vi "MAIN_8.1.vi"() -> ()   [LabVIEW 2013]
doc: "Use this template to build a producer/consumer design pattern with events to produce queue items. Use this design pattern instead of the User Interface Event Handler pattern for user interfaces when you want to execute code asynchronously in response to an event without slowing the user interface responsiveness."
uses:
  State_machine_enum.ctl
  display2.ctl
  User_buttons_enum.ctl
  <vilib>/Analysis/baseanly.llb/Mean (DBL).vi
  <vilib>/DAQmx/read.llb/DAQmx Read (Analog 2D DBL NChan NSamp).vi
  Global 1_diag.vi
  <vilib>/Waveform/WDTFileIO.llb/Export Waveforms To Spreadsheet File (1D).vi
  <vilib>/Utility/file.llb/Write To Spreadsheet File (DBL).vi
  <vilib>/Waveform/WDTFileIO.llb/Export Waveform To Spreadsheet File.vi
  <vilib>/DAQmx/create/channels.llb/DAQmx Create Channel (AI-Voltage-Basic).vi
  <vilib>/DAQmx/configure/timing.llb/DAQmx Timing (Sample Clock).vi
  <vilib>/DAQmx/miscellaneous.llb/DAQmx Fill In Error Info.vi
  <vilib>/express/express arith-compare/Formula/XNode/ExpressFormulaBlockNode.xnode
  <vilib>/Analysis/NI_AALBase.lvlib
  <resource>/objmgr/daqmx.rc
panel:
  out "1f PEM Y":dbl
  out "2f PEM Y":dbl=0.004981012167818904
  out "2f PEM X":dbl=0.004981012167818904
  out "1f PEM X":dbl
  out "2f Spectrum array":dbl[](array[numeric])
  in  "QuickDiag":bool=TRUE
  out "x/y":dbl=0.002005684477504462
  in  "Motor Voltage (V) 2":dbl=1.0 min=0.0 max=9.0
  in  "Time Resolved":bool=TRUE
  in  "Start time":timestamp=timestamp(-9593251199.274853 s since 1904-01-01)
  in  "Timer Start":bool
  out "path":path=path "C:/Users/Adam/Desktop/Diag_Prog_v9/temp.txt"
  in  "Stabilization Time (s)":dbl min=0.0 max=2.0
  out "LD error array disc":dbl[](array[numeric])
  out "LD array disc":dbl[](array[numeric])
  out "result":bool=TRUE
  out "dt":dbl=0.001
  out "dLD_RMS":dbl=-0.0
  out "error out":errorcluster
  out "Unbalanced?":bool
  out "Signal Balance":bool
  out "DC Voltage (V) 2":dbl(knob)=0.000879695520089483 scale=0.0..10.0
  out "2f Frequency (Hz)":dbl(knob)=512.4961246512186 scale=0.0..150.0
  in  "Voltage Divider (10)":bool
  out "Actual Task":string="Processing signal"
  out "Motor Voltage (V)":dbl=1.0
  in  "Initial Voltage (V)":dbl=0.35 min=0.0 max=9.0
  in  "Final Voltage (V)":dbl=0.8 min=0.0 max=2.0
  in  "Voltage Step (V)":dbl=0.065 min=0.0 max=1000.0
  in  "Motor Stabilization Time (s)":dbl(knob)=10.0 step=0.001 scale=0.0..30.0
  out "Initial Voltage (V) 2":dbl=1.0 min=0.0 max=9.0
  in  "Final Voltage (V) 2":dbl=1.4 min=0.0 max=2.0
  in  "Voltage Step (V) 2":dbl=0.1 min=0.0 max=1000.0
  in  "Comment (sample no)":string
  in  "Stop Measurement":bool
  in  "Start Measurement Button":bool
  out "Measurement File":path=path "C:/Users/Adam/Desktop/Diag_Prog_v9/testt"
  in  "New File":bool
  out "Reset?":bool=TRUE
  out "Actual State":T1=enum."Process"
  in  "Tab Control":T2(tab)
  out "Measured Points":T3 format="%0.3f"
  out "Ready?":bool
  out "Ready?":string="Ready?"
  out "Motor":bool=TRUE
  out "Motor":string="Motor: OK"
  out "Quick Status 5":string
  out "Down 2":bool
  out "Up 2":bool
  out "Oscilloscope 2":waveform(dbl)[](graph)=[{"t0"=timestamp(0 s since 1904-01-01), "dt"=0.002, "Y"=array[500 elements]}, {"t0"=timestamp(0 s since 1904-01-01), "dt"=0.002, "Y"=array[500 elements]}]
  out "Signal Balance":bool=TRUE
  out "Laser Noise":bool=TRUE
  out "Signal Balance":string="Signal Balance: OK"
  out "Laser Noise":string="Laser Noise: OK"
  in  "Run Quick Diagnostics":bool
  out "Laser Intensity":bool=TRUE
  out "Laser Intensity":string="Laser Intensity: OK"
  out "Delta":T3 format="%0.3f"
  out "Quick Diagnosis":string="?"
  out "Infected?":bool
  out "Detected Signal (mV/V)":T3 format="%0.3f"
  in  "Measure":bool
  out "Signal Spectrum (mVrms/Vdc) 2":cluster{"f0":dbl, "df":dbl, "magnitude":dbl[]}(graph)={"f0"=0.0, "df"=0.05, "magnitude"=[]}
  in  "Convert mld":bool
  in  "Convert parasiteno":bool
  in  "Convert parasitemia":bool
  in  "Convert cc":bool
  out "MLD (mV/V)":dbl=3.234067345901155 format="%#_3g"
  out "SA 1f (mv/V)":dbl=2.8989130211772483
  out "Lock_in (mV/V)":dbl
  out "dLock_in (mV/V)":dbl
  out "dMLD (mV/V)":dbl=1.4958145805121073 format="%#_3g"
  out "Phase (deg)":dbl=0.5117629371467104 format="%0.2f"
  out "Phase  dev (deg)":dbl=-1.4797919911802346 format="%0.2f"
  out "SA 2f (mv/V)":dbl=4.7886484733621755
  out "MLD Amplitude (mV/V)":cluster{dbl[], dbl[]}(graph)={[811.3544417222341, 811.3544417222341, 811.3544417222341, 812.123069024086, 812.123069024086, 812.123069024086, 812.8874794085821, 812.8874794085821, 812.8874794085821], [1.2454269974542926, 0.5310286252314307, nan, 2.0283944559953087, 0.629318419816088, nan, 4.729881926413262, 1.7382527653890476, nan]}
  in  "dT/T (%)":dbl
  in  "Dilution":dbl=20.0
  in  "Undiluted cc.\n (ng/ml)":dbl
  in  "Undiluted \nParasitemia (%)":dbl format="%#_6f"
  in  "Parasites/ul\nof Blood":dbl
  in  "Convert dT":bool
  in  "MLD (mV/V)":dbl
  out "mean MLD (mV/V)":T3 format="%0.3f"
  out "Delta MLD":T3 format="%0.3f"
  out "DC (V)":cluster{dbl[], dbl[]}(graph)={[811.3544417222341, 812.123069024086, 812.8874794085821], [0.0013390360406046716, 0.001032809026927879, 0.0011348846981534767]}
  out "MLD Phase":cluster{dbl[], dbl[]}(graph)={[811.3544417222341, 811.3544417222341, 811.3544417222341, 812.123069024086, 812.123069024086, 812.123069024086, 812.8874794085821, 812.8874794085821, 812.8874794085821], [3.334514079178165, 1.9138777094600323, nan, 1.9127445130109195, 0.49437453619101257, nan, nan, nan, nan]}
  out "Down":bool
  out "Up":bool
  out "2f Frequency (Hz)":T3=23.056300268096514 format="%0.3f"
  out "1f SA (mV/V)":T3=153.49895465158366 format="%0.3f"
  out "MLD Sim. LIA (mV/V)":T3=nan format="%0.3f"
  out "MLD SA (mV/V)":T3=37.38207236557522 format="%0.3f"
  in  "Start Scope":bool
  in  "Constant Motor Voltage":dbl=1.0 min=0.0 max=3.0
  in  "Refresh in (s)":i8=10
  in  "stop":bool
  in  "AC?":bool
  out "levelB":dbl=0.1 format="%#_2g"
  out "levelA":dbl format="%#_3g"
  in  "V/div B":dbl(knob)=0.2 scale=10.0..0.01 scale format="%#_3g"
  in  "level B":dbl(slide)=0.4 scale=-1.0..1.0 scale format="%#_3g"
  in  "level A":dbl(slide) scale=-1.0..1.0 scale format="%#_3g"
  in  "V/div A":dbl(knob)=0.05 scale=10.0..0.01 scale format="%#.3f"
  out "Oscilloscope":waveform(dbl)[](graph)=[{"t0"=timestamp(0 s since 1904-01-01), "dt"=0.0025, "Y"=array[375 elements]}, {"t0"=timestamp(0 s since 1904-01-01), "dt"=0.0025, "Y"=array[375 elements]}]
  in  "Sensitivity":T4(ring)
  in  "samples per channel":i32=1000
  in  "rate":dbl=1000.0 format="%0.2f"
  out "Spectrum (mVRMS/Vdc)":cluster{"f0":dbl, "df":dbl, "magnitude":dbl[]}(graph)={"f0"=0.0, "df"=1.0, "magnitude"=[1338.0484216778725, 891.4717650116102, 143.2192215595614, 172.79898091711885, 95.50453001628563, 113.23096269717587, 159.9728459536367, 142.17510842649094, 23.555096842939967, 172.4586840116519, 233.3391086271948, 153.49895465158366, 59.303017218056304, 51.41913744169332, 87.60985790792097, 89.15548748523767, 102.41083253503767, 116.69415211742178, 102.04780407888852, 98.07941394008398, 62.015801498942174, 57.365633541451224, 37.38207236557522, 140.01194138717574, 88.85968438008766, 51.8911573784031, 96.44625566359282, 102.80626369349147, 154.32416325374467, 152.72565881880075, 63.97627104136422, 44.061183722532256, 24.299532372372934, 66.51944362511281, 119.45636901763923, 79.60274206424093, 126.46507446936278, 115.56735495111872, 86.92439368676867, 42.47483057858276, 45.987972767001125, 82.38613913097223, 57.14235729256332, 24.715704736492583, 91.95786457200892, 229.45656360476565, 301.7932887816684, 181.94479488218664, 9.707170408716356, 79.16705422107816, 32.4671901662433, 34.994674897672475, 45.603676560961965, 81.17087782317107, 123.48392300390853, 125.53549820312338, 197.71297955832767, 51.56670220175255, 139.4897349387358, 136.00021553543283, 49.84751230386803, 106.388211919061, 128.21302631973177, 179.83380975700697, 238.686425101159, 204.64888147263136, 159.4400865495827, 88.9566203515302, 50.82386237011203, 47.10090178269198, 31.249556983451996, 155.07366739734923, 197.20488460315576, 181.86491698592144, 122.60135896300172, 15.723508058553668, 47.32988919426525, 91.09235604990127, 70.08764782926058, 71.11042986773145, 167.58334514547386, 157.0684001711449, 85.4088975978964, 165.68125229281705, 108.34787076535925, 58.32465184772515, 102.85811162079386, 88.031264754637, 35.99088343784742, 74.99228300753498, 59.59436041355427, 109.74543517855098, 239.92689639368845, 195.22681808589817, 153.93792803433803, 171.35120542643082, 103.04216715301814, 144.22424620891795, 33.236928017526, 33.6474288996255, 71.18496484217899, 175.10446025244616, 221.24997378317522, 114.75466832528755, 52.3833439055373, 114.90211538243959, 94.87498722211751, 82.82924122532899, 124.12586199482064, 107.6258638888207, 78.5024563400891, 92.06245924719637, 16.228987466475928, 84.84217000760313, 88.76503911599063, 114.25618103440272, 155.27289903749065, 116.20062823456668, 61.96139303164934, 214.19314697712042, 248.12058486418763, 215.9112937618697, 145.04293815290015, 142.16464369485132, 169.7377761460246, 83.55657324380019, 74.4879617799582, 39.81106304135121, 152.2410798694005, 176.4879867987291, 110.01229615691923, 89.83888006443468, 195.69702436303007, 166.19892376632072, 55.02836867851484, 113.06515146784245, 221.3685360221306, 181.10055208661387, 262.0371181638539, 185.73443857709046, 93.90961856721144, 84.54783744027858, 24.449872475327695, 95.3789149136639, 140.24246950513043, 143.73337464437884, 33.58378655631947, 62.839362697344995, 57.47449635929643, 139.96968907631262, 167.0231838520772, 135.6723918020847, 124.14523269479409, 111.37946391963057, 195.70470757666732, 192.9947832776428, 93.91006382282066, 121.56931305302999, 113.63589006917633, 42.92804035457153, 141.48803985115433, 165.5507518379778, 121.34962379960878, 143.04362518480343, 22.72432951654588, 183.17549468524615, 152.95042171438013, 195.3079831947777, 131.83171839040367, 30.49881104219535, 8.46043248589554, 141.40803256070282, 223.72992955634092, 132.30059550265176, 54.60897309407436, 84.56504745319246, 125.72411835874722, 194.72474433717994, 126.94182365881618, 27.456941187399302, 114.85067679816903, 138.3914927403539, 237.22038521157256, 172.58040690453, 178.93819766022105, 171.11586449112946, 66.32529189912087, 175.61268977844438, 179.0727535154661, 223.71442469320746, 230.52161416220554, 181.0440521026372, 72.70233235363926, 157.99312186800248, 143.29067791998708, 138.45794114882568, 122.15383561979628, 55.90884824057415, 43.2895289444191, 25.99180252149831]}
  out "MLD LIA (mV/V)":dbl=0.0123978
  out "Lockin_freq":dbl=9.4676
  out "DC Voltage (V)":T3=0.000879695520089483 format="%0.3f"
  out "Time Domain Signal":cluster{"xi used":dbl[], "yi":dbl[]}[](graph)
  out "Signal Spectrum (mVrms/Vdc)":cluster{"f0":dbl, "df":dbl, "magnitude":dbl[]}[](graph)=[{"f0"=0.0, "df"=0.049999500004999954, "magnitude"=array[50001 elements]}, {"f0"=0.0, "df"=0.05, "magnitude"=array[5000 elements]}]
  out "1f 2f Spectral Peaks":T5={"1f (Hz)"=256.112805640282, "U1f (mV/V)"=2.8989130211772483, "2f (Hz)"=512.375618780939, "U2f (mV/V)"=4.7886484733621755}
  out "LockIN Theta (cont/disc)":waveform(dbl)(graph)={"t0"=timestamp(0 s since 1904-01-01), "dt"=0.002, "Y"=array[5000 elements]}
  out "LockIN R (cont/disc)":waveform(dbl)(graph)={"t0"=timestamp(0 s since 1904-01-01), "dt"=0.002, "Y"=array[5000 elements]}
  out "Lockin R":waveform(dbl)(graph)
  out "Lockin Theta":waveform(dbl)(graph)
  out "2f PEM R":dbl=0.004981012167818904
  out "1f PEM R":dbl
  out "PEM spectrum":cluster{"f0":dbl, "df":dbl, "magnitude":dbl[]}(graph)
  out "Lockin X,Y,R":waveform(dbl)[](graph)
  out "PEM spectrum X,Y,R":cluster{"f0":dbl, "df":dbl, "magnitude":dbl[]}[](graph)
  in  "Pike Removal (StDev)":dbl=3.0
  in  "Lock-in Time (s)":dbl=10.0
  in  "dt (s)":dbl=0.0002
  in  "Resolution (s)":dbl=0.0001
  in  "Averaging time (s)":dbl=1.0 format="%0.2p"
  in  "Cutoff Frequency (Hz)":dbl=500.0
  in  "Rate":dbl=5000.0 caption="Sample Rate (Hz)" format="%0.2f"
  in  "Samples per Channel":i32=100000
  out "Minimum Value":dbl=-1.0 caption="LD min Value (V)" format="%0.2f"
  out "Maximum Value":dbl=1.0 caption="LD max Value (V)" format="%0.2f"
  in  "DC # samples":i32=100
  in  "DC Sampling Rate (Hz)":dbl=100.0
  in  "Dc min":dbl format="%0.2f"
  in  "Dc max":dbl=10.0 format="%0.2f"
  in  "Reference Signal":tag="Dev2/ai3"
  in  "LD Signal":tag="Dev2/ai0" caption="LD Channel"
  in  "DC Voltage DAQ":tag="Dev2/ai1"
  in  "Motor Channel":tag="Dev2/ao0"
  in  "Lock-in-Amplifier VISA":refnum<visa-resource-name>="GPIB0::3::INSTR"
  in  "Second Harmonic":bool
  in  "Lock In":bool
  in  "Continous Lock-in":bool=TRUE
  in  "LockIn":bool
  in  "Save graphs":bool
  out "Dc standard deviation":dbl=0.002551891780639937 format="%0.2f"
  out "Dc mean":dbl=0.000879695520089483 format="%0.2f"
  out "dPhase array":dbl[](array[numeric])=[0.7103181848590662, 0.7091849884099535, 0.5117629371467104]
  out "Phase array":dbl[](array[numeric])=[2.6241958943190986, 1.203559524600966, nan, 1.2024263281518537, -0.21594364866805338, nan, -1.4797919911802346]
  out "LD array":dbl[](array[numeric])=[0.8882278113428617, 1.3288564379056984, 3.234067345901155]
  out "Frequency array":dbl[](array[numeric])=[811.3544417222341, 812.123069024086, 812.8874794085821]
  out "LD error array":dbl[](array[numeric])=[0.357199186111431, 0.6995380180896104, 1.4958145805121073]
  out "First?":bool
  out "Stopped":bool
  out "Last Step?":bool
  in  "EXIT":bool
  # "Measurement Settings"
  # "Motor Setup"
  # "OFF"
  # "ON"
  # "Setup"
  # "Status:"
  # "Measurement"
  # "mV/V"
  # "±"
  # "Detected Magneto-Optical Signal:"
  # "Quick Diagnosis Report:"
  # "Measured points:"
  # "Actual Datapoint Values"
  # "mV/V"
  # "±"
  # "Convert quantities"
  # "Physical channels"
  # "Signal Processing Settings"
  # "DC Acquisition Settings"
  # "LD Acquisition Settings"
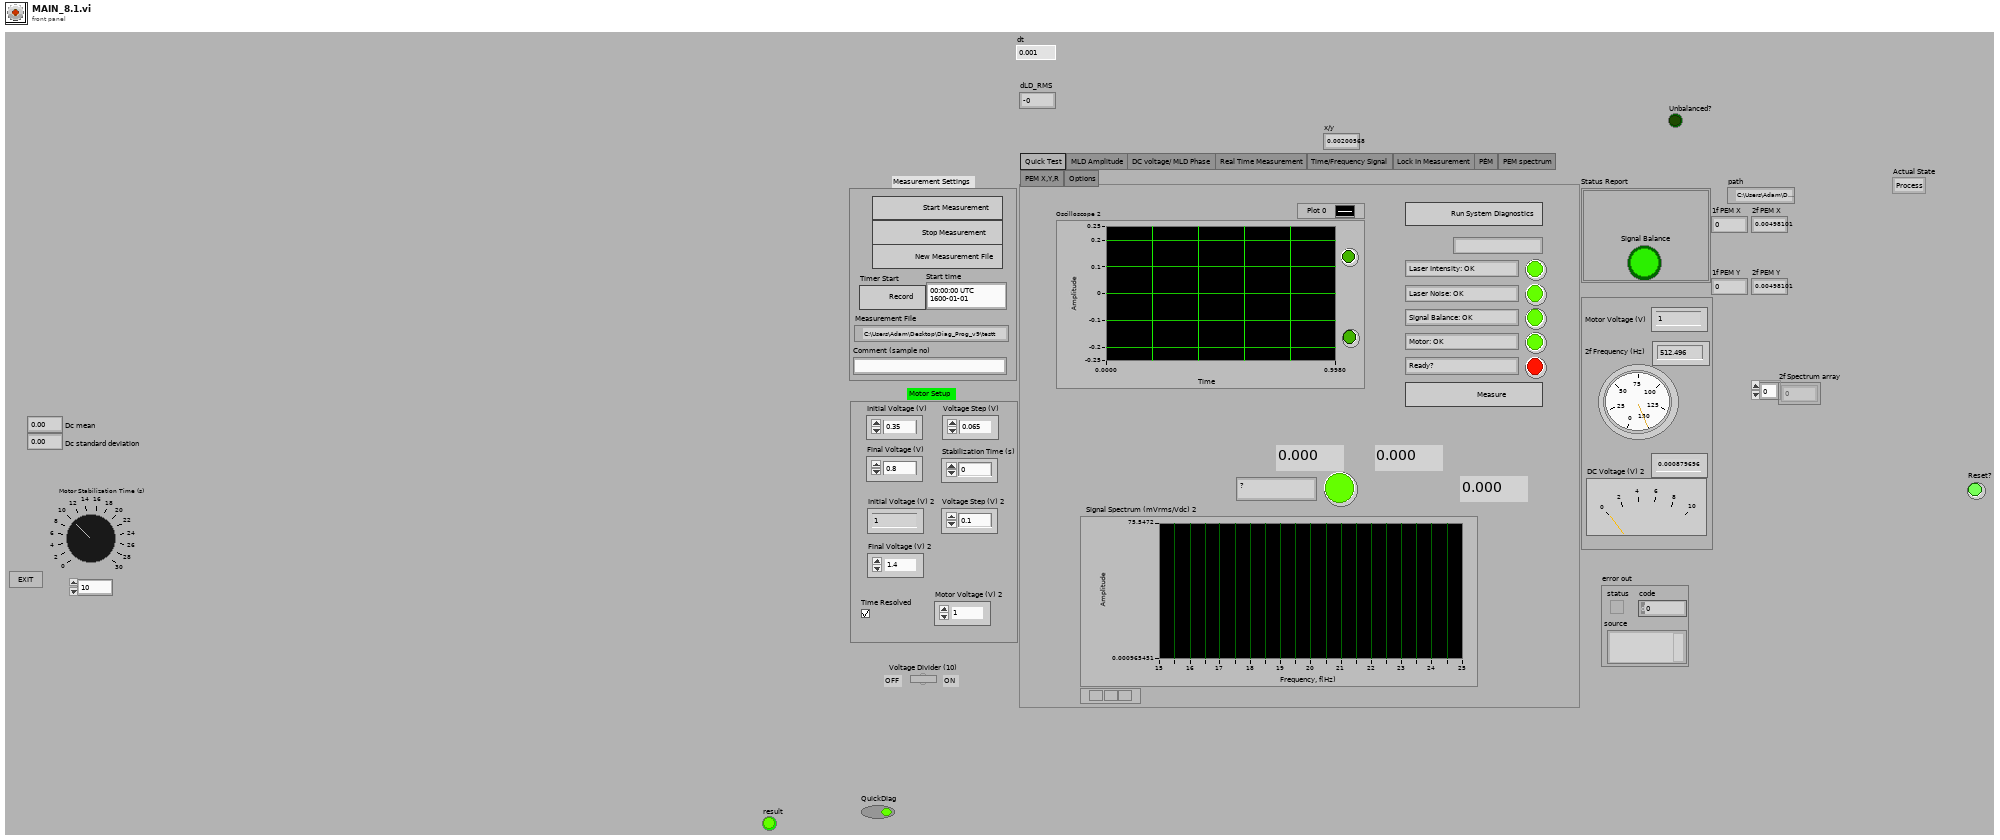
[diagram p1: front panel]
types:
  T1 = typedef "State_machine_enum.ctl" = enum16{"SetMotor", "Stabilize", "Measure", "Process", "Save", "Finished"}
  T2 = enum32{"Quick Test", "MLD Amplitude", "DC voltage/ MLD Phase", "Real Time Measurement", "Time/Frequency Signal", "Lock In Measurement", "PÉM", "PEM spectrum", "PEM X,Y,R", "Options"}
  T3 = typedef "display2.ctl" = dbl
  T4 = enum16{"-1V..1V", "-1.25V..1.25V", "-2V..2V", "-2.5V..2.5V", "-4V..4V", "-5V..5V", "-10V..10V"}
  T5 = cluster{"1f (Hz)":dbl, "U1f (mV/V)":dbl, "2f (Hz)":dbl, "U2f (mV/V)":dbl}
  T6 = typedef "User_buttons_enum.ctl" = enum16{"start", "stop", "exit", "New", "Scope", "Continue"}
  T7 = enum16{"open", "replace", "create", "open or create", "replace or create", "replace or create with confirmation"}
  T8 = enum8{"Enabled", "Disabled", "Disabled and Grayed Out"}
  T9 = enum16{"Left Button", "Center Button", "Right Button", "Window Close"}
  T10 = cluster{dbl, "1f Ampl (Vrms/Vdc)":dbl, dbl, "2f Ampl (Vrms/Vdc)":dbl}
  T11 = cluster{"MLD":dbl, "dMLD":dbl, "Phase":dbl, "dPhase":dbl}
  T12 = cluster{"Frequency array":dbl[], "LD array":dbl[]}
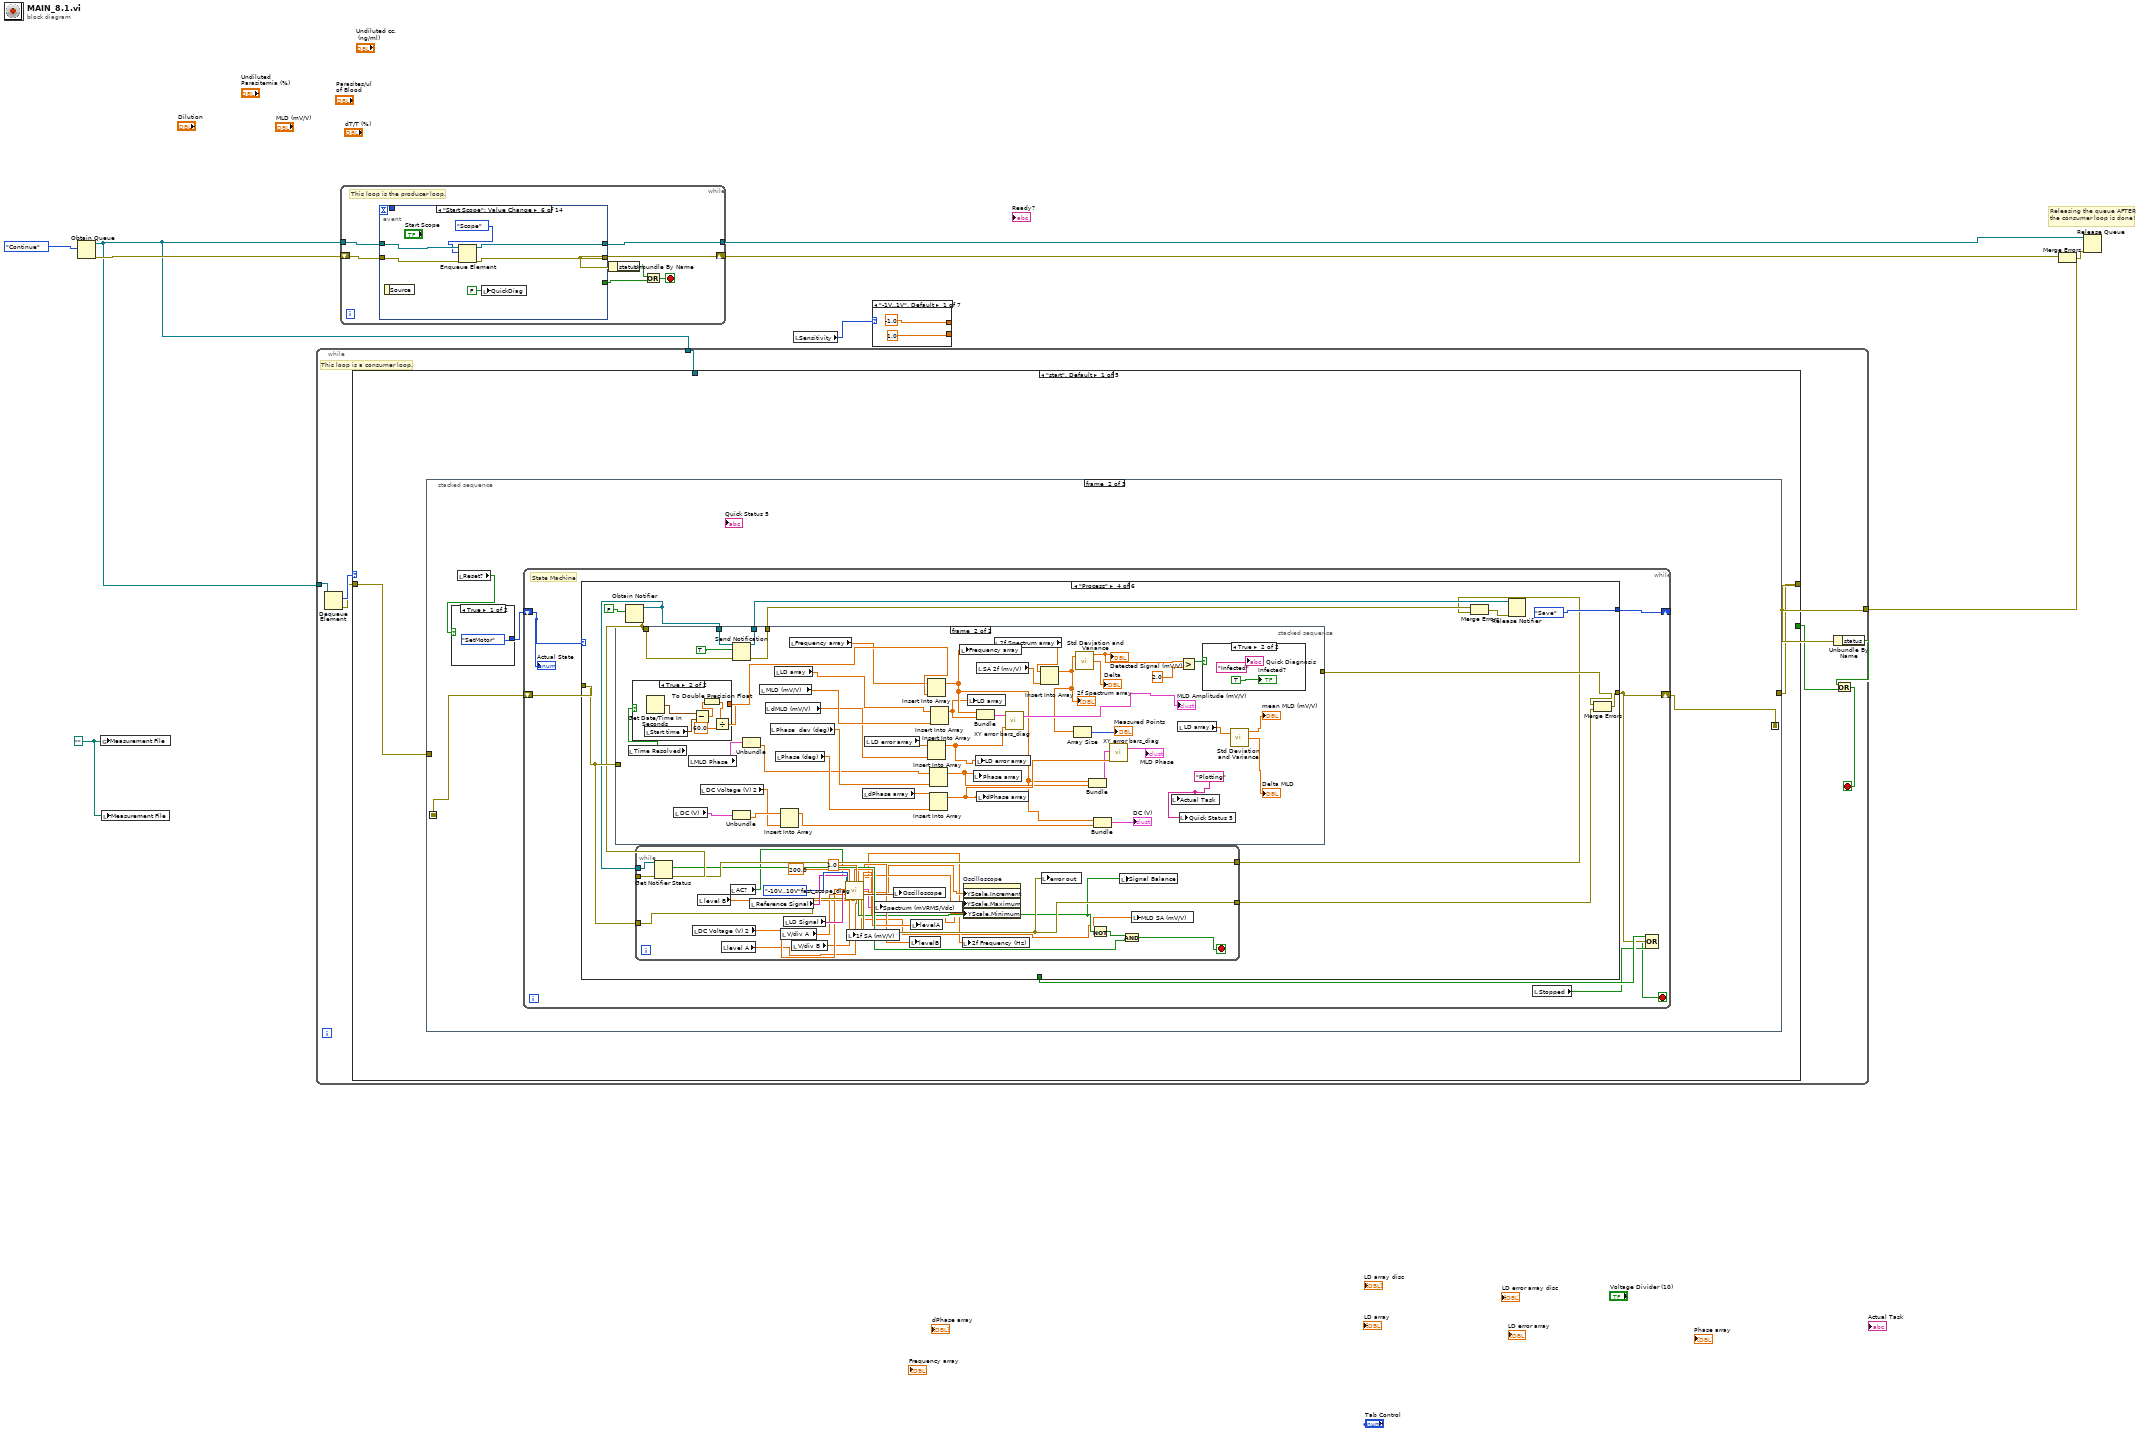
[diagram p0: block diagram]
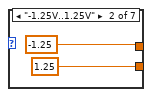
[diagram p2: hidden frame]
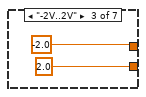
[diagram p3: hidden frame]
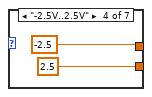
[diagram p4: hidden frame]
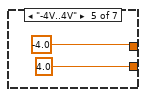
[diagram p5: hidden frame]
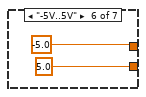
[diagram p6: hidden frame]
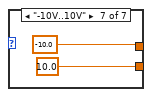
[diagram p7: hidden frame]
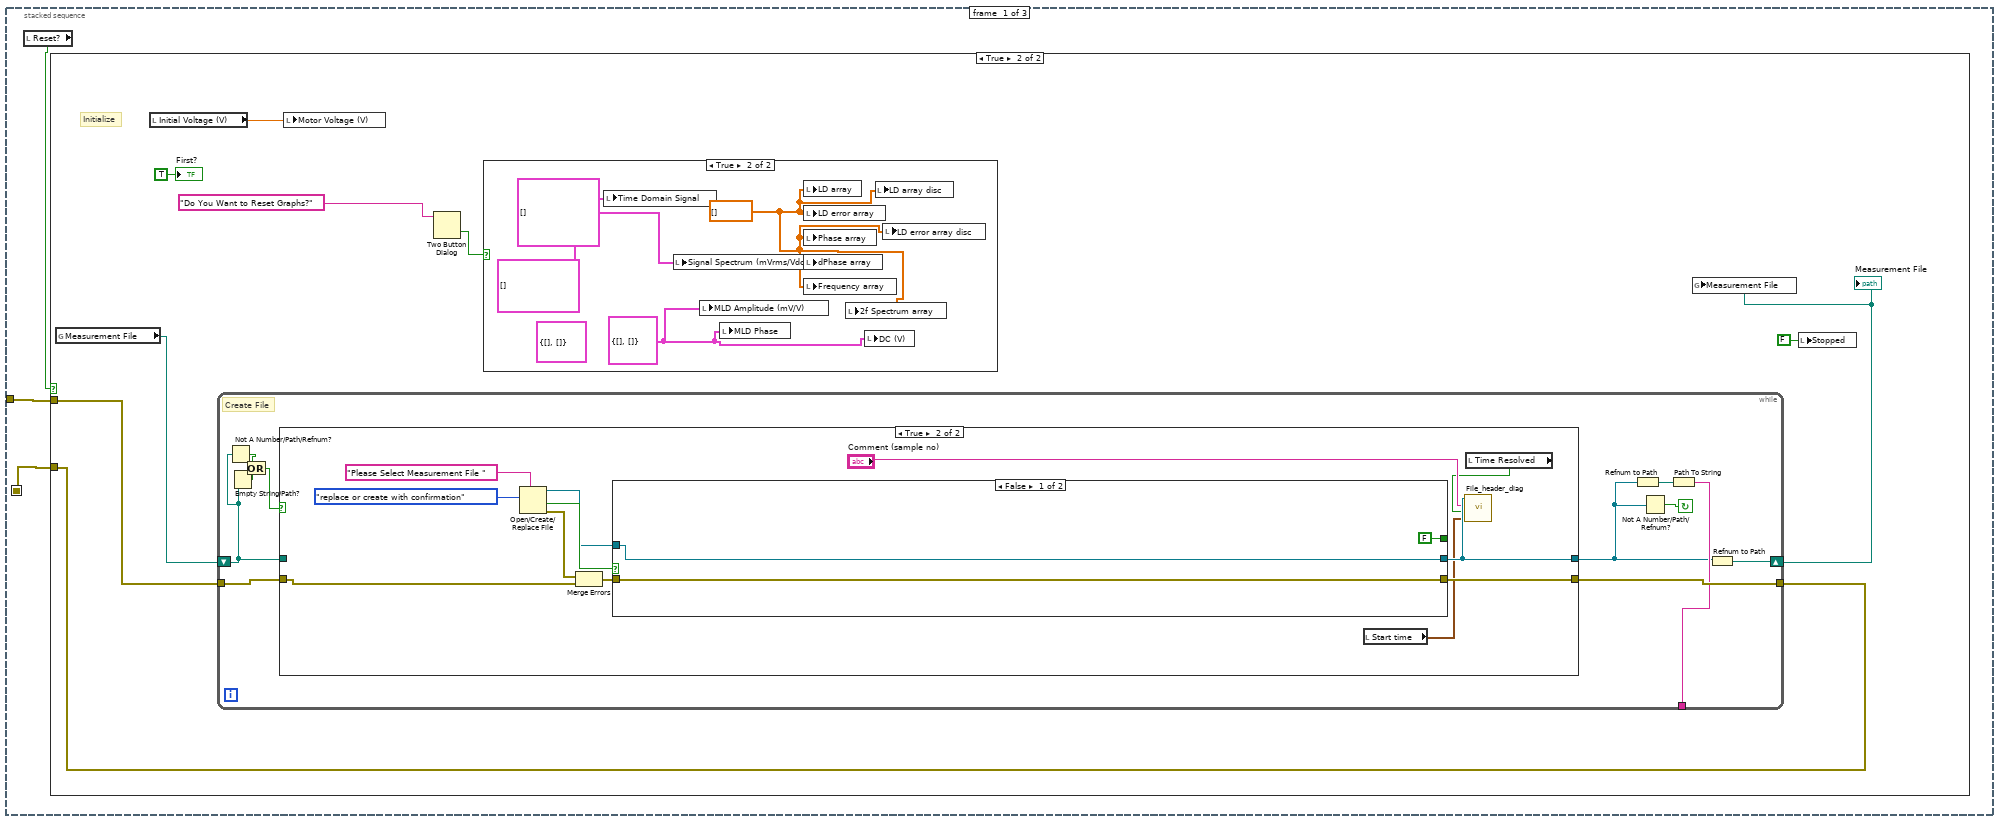
[diagram p8: hidden frame]
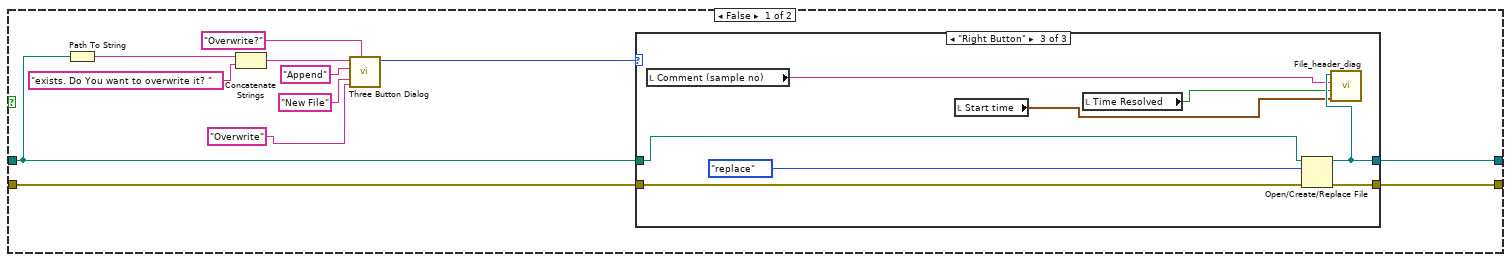
[diagram p10: hidden frame]
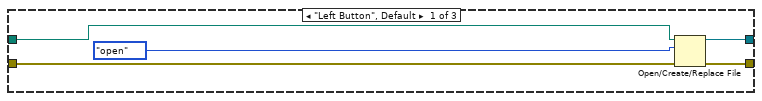
[diagram p11: hidden frame]
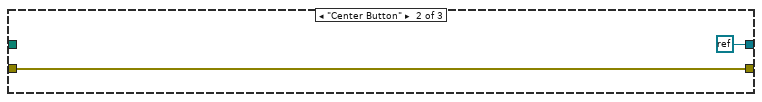
[diagram p12: hidden frame]
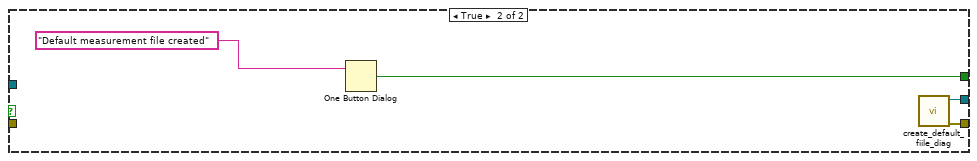
[diagram p13: hidden frame]
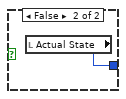
[diagram p15: hidden frame]
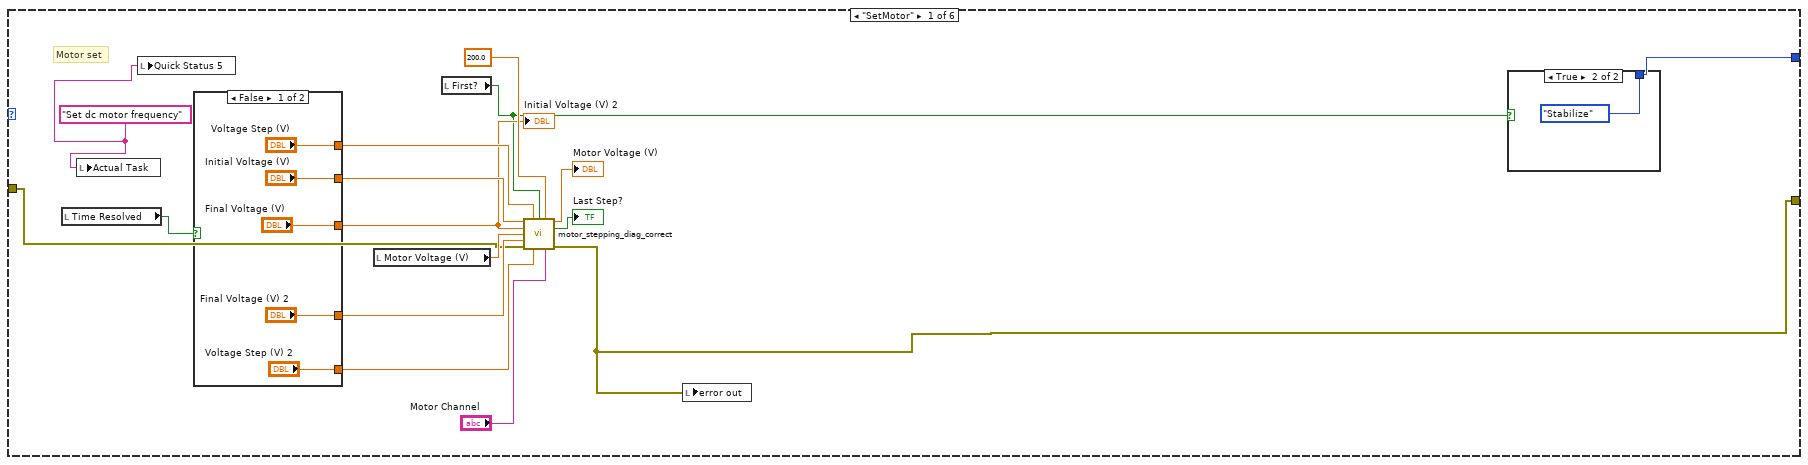
[diagram p16: hidden frame]
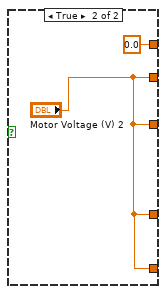
[diagram p17: hidden frame]
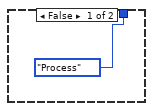
[diagram p18: hidden frame]
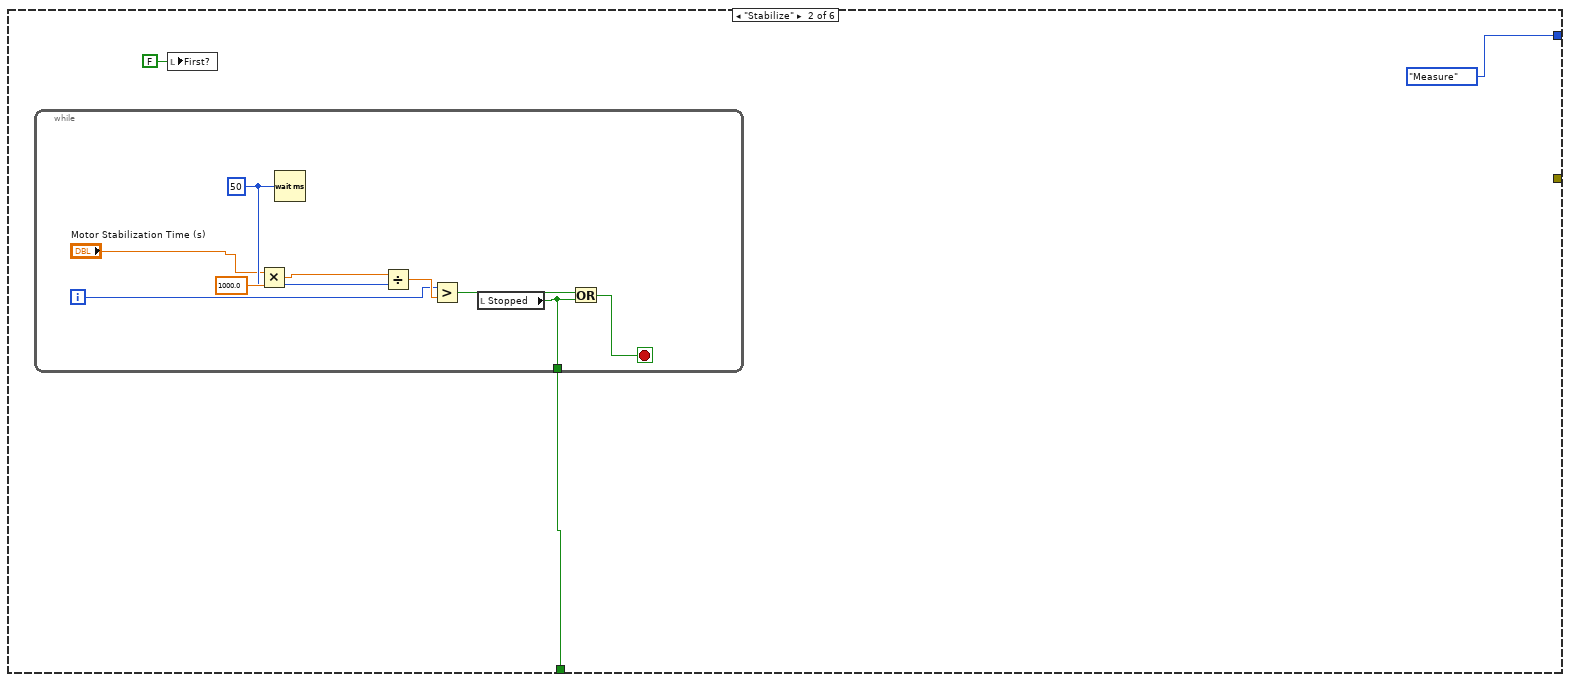
[diagram p19: hidden frame]
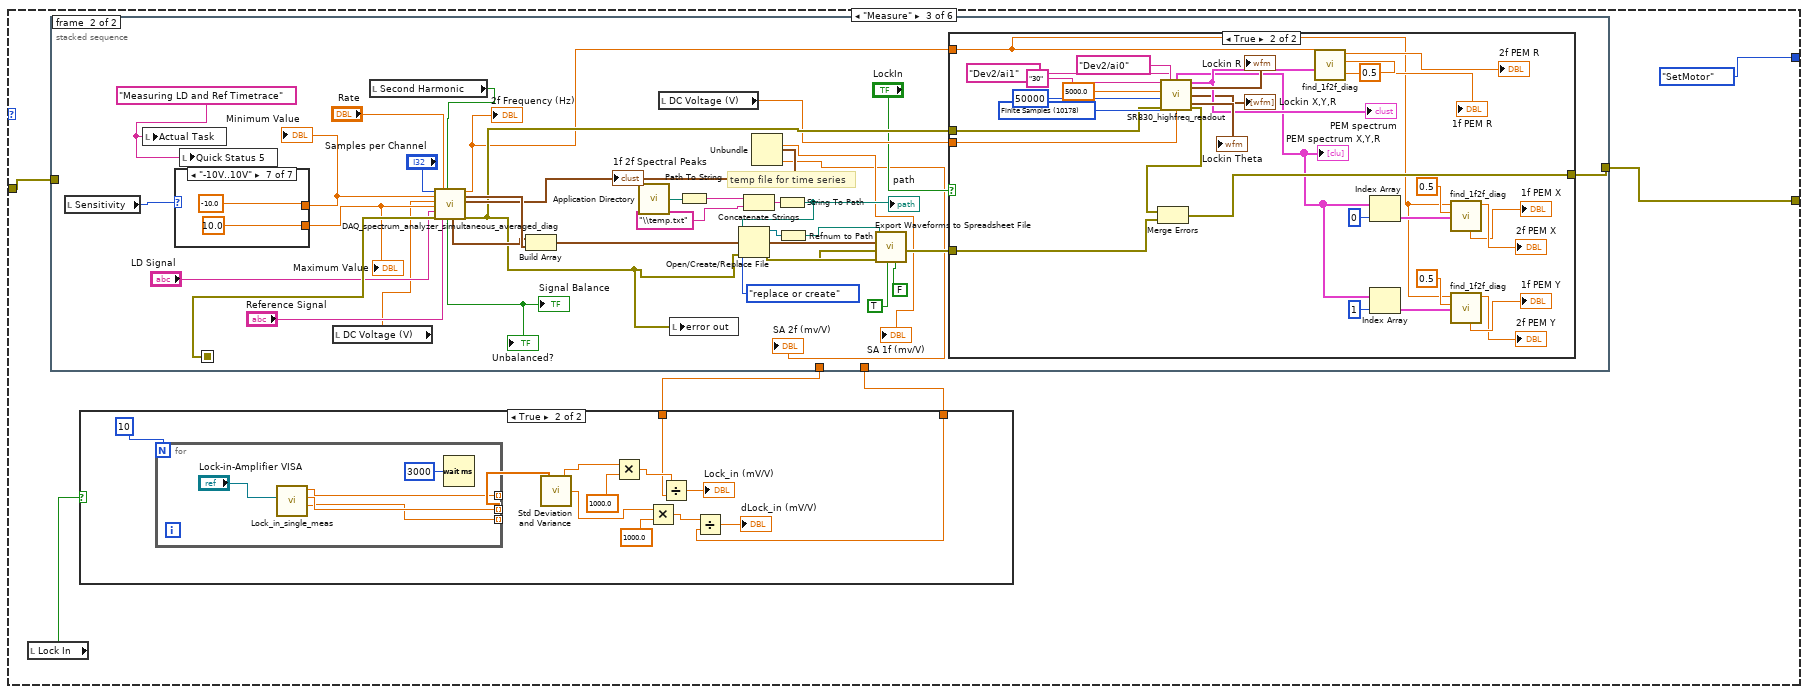
[diagram p20: hidden frame]
diagram:
  w1 = path ""
  # "Releasing the queue AFTER\nthe consumer loop is done!"
  n1 = Obtain Queue(element data type=User_buttons_enum."Continue") -> (queue out=w3:refnum<queue>, error out=w9:errorcluster)  [unwired: 4 in, 1 out]
  n2 = global write "Global 1_diag.vi" "Measurement File"(w1) -> ()
  n3 = local write "Measurement File"(w1) -> ()
  n4 = while {
    tunnel: w3 -> [w17]
    tunnel: [w14] -> w5
    tunnel: w3 -> [w10]
    stop <- w11 stop-if-true
    # "This loop is a consumer loop."
    n5 = Dequeue Element(queue=w17) -> (element=w16:T6, error out=w15:errorcluster)  [unwired: 2 in, 2 out]
    n6 = case shown="\"start\", Default" w16 {
      tunnel: [_ _ TRUE _ _] -> w12
      tunnel: w15 -> [w19 w499 w561 w565 w575]
      tunnel: [w18 w498 w561 w564 w581] -> w14
      tunnel: w10 -> [_ w497 _ _ w567]
      frame "start", Default {
        n7 = stacked-sequence {
          seq-local: [w21 _ _] -> [_ w97 _]
          seq-local: [_ w96 _] -> [_ _ w484]
          tunnel: w19 -> [w22 _ w482]
          tunnel: [_ _ w481] -> w18
          frame #0 {
            n8 = local read "Reset?"() -> (w20:bool)
            n9 = case shown="True" w20 {
              tunnel: w22 -> [w23 w27]
              tunnel: [w23 w25] -> w21
              frame False {
              }
              frame True {
                # "Initialize"
                n10 = global read "Global 1_diag.vi" "Measurement File"() -> (w26:path)
                n11 = local read "Initial Voltage (V)"() -> (w30:dbl)
                n12 = while {
                  tunnel: [w43] -> w25
                  tunnel: w27 -> [w42]
                  shift-right: [w37] -> w24
                  shift-left: w26 -> [w36]
                  tunnel: [w39] -> _
                  stop <- w41 continue-if-true
                  # "Create File"
                  n13 = Not A Number/Path/Refnum?(number/path/refnum=w36) -> (NaN/Path/Refnum?=w35:bool)
                  n14 = Empty String/Path?(string/path=w36) -> (empty?=w34:bool)
                  n15 = Or(x=w35, y=w34) -> (x .or. y?=w33:bool)
                  n16 = case shown="True" w33 {
                    tunnel: [w50 w75] -> w38
                    tunnel: [w49 w74] -> w43
                    tunnel: w42 -> [w48 w76]
                    tunnel: w36 -> [w44 _]
                    frame False {
                      n17 = Path To String(path=w44) -> (string=w47:string)
                      n18 = Concatenate Strings(w47, "exists. Do You want to overwrite it? " ("message")) -> (w45:string)
                      n19 = call <vilib>:"Three Button Dialog.vi"("Window Title (\"\")"="Overwrite?" ("Window Title (\"\")"), "Right Button Text (\"Cancel\")"="Overwrite" ("Right Button Text (\"Cancel\")"), "Center Button Text (\"No\")"="New File" ("Center Button Text (\"No\")"), "Left Button Text (\"Yes\")"="Append" ("Left Button Text (\"Yes\")"), "message"=w45) -> ("Which Button?"=w51:T9)  [unwired: 6 in]
                      n20 = case shown="\"Right Button\"" w51 {
                        tunnel: w44 -> [w56 _ w66]
                        tunnel: [w57 refnum<k0> refnum w67] -> w50
                        tunnel: [w59 w61 w69] -> w49
                        tunnel: w48 -> [w58 w61 w68]
                        frame "Left Button", Default {
                          n21 = Open/Create/Replace File(file path (use dialog)=w56, error in=w58, operation (0:open)=T7."open") -> (refnum out=w57:refnum<file>, error out=w59:errorcluster)  [unwired: 3 in, 1 out]
                        }
                        frame "Center Button" {
                        }
                        frame "Right Button" {
                          n22 = local read "Comment (sample no)"() -> (w65:string)
                          n23 = local read "Start time"() -> (w63:timestamp)
                          n24 = local read "Time Resolved"() -> (w64:bool)
                          n25 = Open/Create/Replace File(file path (use dialog)=w66, error in=w68, operation (0:open)=T7."replace") -> (refnum out=w67:refnum<file>, error out=w69:errorcluster)  [unwired: 3 in, 1 out]
                          n26 = call "File_header_diag.vi"("Preparation time"=w63, "Time resolved?"=w64, "Comment"=w65, "Byte Stream File in"=w67) -> ()  [unwired: 8 in]
                        }
                      }
                    }
                    frame True {
                      n27 = Open/Create/Replace File(prompt="Please Select Measurement File ", operation (0:open)=T7."replace or create with confirmation") -> (refnum out=w79:refnum<file>, cancelled=w80:bool, error out=w78:errorcluster)  [unwired: 4 in]
                      n28 = Merge Errors(w78, w76) -> (w77:errorcluster)
                      n29 = case shown="False" w80 {
                        tunnel: w79 -> [w85 _]
                        tunnel: [w85 w86] -> w75
                        tunnel: [w84 w88] -> w74
                        tunnel: w77 -> [w84 _]
                        tunnel: [FALSE ("true") w87] -> _
                        frame False {
                        }
                        frame True {
                          n30 = One Button Dialog(message="Default measurement file created") -> (true=w87:bool)  [unwired: 1 in]
                          n31 = call "create_default_fiile_diag.vi"() -> ("error out"=w88:errorcluster, "Byte Stream File out"=w86:refnum<file>)  [unwired: 10 in]
                        }
                      }
                      n32 = local read "Start time"() -> (w71:timestamp)
                      n33 = local read "Time Resolved"() -> (w72:bool)
                      n34 = call "File_header_diag.vi"("Preparation time"=w71, "Time resolved?"=w72, "Comment"="Comment (sample no)", "Byte Stream File in"=w75) -> ()  [unwired: 8 in]
                    }
                  }
                  n35 = Refnum to Path(1:w38) -> (0:w40:path)
                  n36 = Not A Number/Path/Refnum?(number/path/refnum=w38) -> (NaN/Path/Refnum?=w41:bool)
                  n37 = Path To String(path=w40) -> (string=w39:string)
                  n38 = Refnum to Path(1:w38) -> (0:w37:path)
                }
                "Measurement File" <- w24
                n39 = local write "Motor Voltage (V)"(w30) -> ()
                n40 = Two Button Dialog(message="Do You Want to Reset Graphs?") -> (T button?=w28:bool)  [unwired: 2 in]
                n41 = case shown="True" w28 {
                  frame False {
                  }
                  frame True {
                    w91 = cluster{dbl[], dbl[]} {[], []} ("MLD Amplitude (mV/V)")
                    (unwired) cluster{"magnitude":dbl[], "magnitude 2":dbl[]} {"magnitude"=[], "magnitude 2"=[]} ("MLD Amplitude")
                    w90 = dbl[] []
                    n42 = local write "Time Domain Signal"(cluster{dbl[], dbl[]}[] [] ("Integral")) -> ()
                    n43 = local write "Signal Spectrum (mVrms/Vdc)"(cluster{"f0":dbl, "df":dbl, dbl[]}[] [] ("Signal Spectrum")) -> ()
                    n44 = local write "MLD Amplitude (mV/V)"(w91) -> ()
                    n45 = local write "MLD Phase"(w91) -> ()
                    n46 = local write "LD array"(w90) -> ()
                    n47 = local write "LD error array"(w90) -> ()
                    n48 = local write "Phase array"(w90) -> ()
                    n49 = local write "dPhase array"(w90) -> ()
                    n50 = local write "Frequency array"(w90) -> ()
                    n51 = local write "2f Spectrum array"(w90) -> ()
                    n52 = local write "DC (V)"(w91) -> ()
                    n53 = local write "LD array disc"(w90) -> ()
                    n54 = local write "LD error array disc"(w90) -> ()
                  }
                }
                n55 = global write "Global 1_diag.vi" "Measurement File"(w24) -> ()
                n56 = local write "Stopped"(FALSE ("Stopped")) -> ()
                "First?" <- TRUE ("First?")
              }
            }
          }
          frame #1 {
            n57 = local read "Reset?"() -> (w94:bool)
            n58 = case shown="True" w94 {
              tunnel: [State_machine_enum."SetMotor" w99] -> w95
              frame True {
              }
              frame False {
                n59 = local read "Actual State"() -> (w99:T1)
              }
            }
            n60 = while {
              shift-right: [w100] -> _
              shift-left: w95 -> [w106]
              shift-right: [w104] -> w96
              shift-left: w97 -> [w101]
              stop <- w102 stop-if-true
              # "State Machine"
              n61 = case shown="\"Process\"" w106 {
                tunnel: [w108 _ w149 w267 w431 _] -> w104
                tunnel: [_ w134 _ _ _ w480] -> w105
                tunnel: w101 -> [w117 _ w148 w265 w431 _]
                tunnel: [w122 State_machine_enum."Measure" State_machine_enum."SetMotor" State_machine_enum."Save" w430 State_machine_enum."SetMotor"] -> w100
                frame "SetMotor" {
                  w107 = "Set dc motor frequency" ("Actual Task")
                  # "Motor set"
                  n62 = local read "Time Resolved"() -> (w109:bool)
                  n63 = local write "Actual Task"(w107) -> ()
                  n64 = local write "Quick Status 5"(w107) -> ()
                  n65 = case shown="False" w109 {
                    tunnel: ["Initial Voltage (V)" "Motor Voltage (V) 2"] -> w121
                    tunnel: ["Final Voltage (V) 2" "Motor Voltage (V) 2"] -> w118
                    tunnel: ["Voltage Step (V)" 0.0 ("Voltage Step (V)")] -> w116
                    tunnel: ["Voltage Step (V) 2" "Motor Voltage (V) 2"] -> w115
                    tunnel: ["Final Voltage (V)" "Motor Voltage (V) 2"] -> w111
                    frame False {
                    }
                    frame True {
                    }
                  }
                  "Initial Voltage (V) 2" <- w111
                  n66 = local read "Motor Voltage (V)"() -> (w119:dbl)
                  n67 = local read "First?"() -> (w110:bool)
                  n68 = call "motor_stepping_diag_correct.vi"("Initial Voltage (V)"=w121, "Voltage Step (V)"=w116, "First?"=w110, "Steps"=200.0, "Final Voltage (V)"=w111, "Actual Voltage (V)  in"=w119, "Final Voltage (V) 2"=w118, "error in (no error)"=w117, "Voltage Step2"=w115, "Physical Channel"="Motor Channel") -> ("Actual Voltage (V)"=→"Motor Voltage (V)":dbl, "Boolean"=→"Last Step?":bool, "error out"=w108:errorcluster)  [unwired: 3 in]
                  n69 = local write "error out"(w108) -> ()
                  n70 = case shown="True" w110 {
                    tunnel: [State_machine_enum."Process" State_machine_enum."Stabilize"] -> w122
                    frame False {
                    }
                    frame True {
                    }
                  }
                }
                frame "Stabilize" {
                  n71 = while {
                    tunnel: [w135] -> w134
                    i -> [w136]
                    stop <- w138 stop-if-true
                    w141 = u32 50 ("milliseconds to wait")
                    n72 = Multiply(x="Motor Stabilization Time (s)", y=1000.0) -> (x*y=w143:dbl)
                    n73 = Wait (ms)(milliseconds to wait=w141) -> ()  [unwired: 1 out]
                    n74 = Divide(x=w143, y=w141) -> (x/y=w140:dbl)
                    n75 = Greater?(x=w136, y=w140) -> (0:w139:bool)
                    n76 = local read "Stopped"() -> (w135:bool)
                    n77 = Or(x=w139, y=w135) -> (x .or. y?=w138:bool)
                  }
                  n78 = local write "First?"(FALSE ("First?")) -> ()
                }
                frame "Measure" {
                  n79 = local read "Lock In"() -> (w144:bool)
                  n80 = stacked-sequence {
                    seq-local: [w173 _] -> [_ w213]
                    tunnel: [_ w184] -> w149
                    tunnel: w148 -> [w169 _]
                    tunnel: [w168 _] -> w147
                    tunnel: [w168 _] -> w146
                    frame #0 {
                      w167 = "Measuring DC Voltage" ("Actual Task")
                      n81 = local write "Actual Task"(w167) -> ()
                      n82 = local write "Quick Status 5"(w167) -> ()
                      n83 = call "manualDAQ_diag.vi"("minimum value"="Dc min", "Rate"="DC Sampling Rate (Hz)", "error in (no error)"=w169, "Samples per Channel"="DC # samples", "maximum value"="Dc max", "physical channels"="DC Voltage DAQ") -> ("error out"=w173:errorcluster, "output waveform"=w175:waveform(dbl))  [unwired: 4 in]
                      "error out" <- w173
                      n84 = Unbundle By Name(w175) -> ("Y"=w176:dbl[])
                      n85 = call <vilib>:"Std Deviation and Variance.vi"("X"=w176) -> ("mean"=w168:dbl, "standard deviation"=→"Dc standard deviation":dbl)  [unwired: 1 in, 1 out]
                      "DC Voltage (V) 2" <- w168
                      "Dc mean" <- w168
                      n86 = local write "DC Voltage (V)"(w168) -> ()
                    }
                    frame #1 {
                      w187 = "Measuring LD and Ref Timetrace" ("Actual Task")
                      # "temp file for time series"
                      n87 = local read "Sensitivity"() -> (w201:T4)
                      n88 = local write "Actual Task"(w187) -> ()
                      n89 = case shown="\"-10V..10V\"" w201 {
                        tunnel: [-1.0 ("maximum value") -1.25 ("maximum value") -2.0 ("maximum value") -2.5 ("maximum value") -4.0 ("maximum value") -5.0 ("maximum value") -10.0 ("maximum value")] -> w200
                        tunnel: [1.0 ("maximum value") 1.25 ("maximum value") 2.0 ("maximum value") 2.5 ("maximum value") 4.0 ("maximum value") 5.0 ("maximum value") 10.0 ("maximum value")] -> w199
                        frame "-1V..1V", Default {
                        }
                        frame "-1.25V..1.25V" {
                        }
                        frame "-2V..2V" {
                        }
                        frame "-2.5V..2.5V" {
                        }
                        frame "-4V..4V" {
                        }
                        frame "-5V..5V" {
                        }
                        frame "-10V..10V" {
                        }
                      }
                      "Maximum Value" <- w199
                      "Minimum Value" <- w200
                      n90 = local write "Quick Status 5"(w187) -> ()
                      n91 = local read "DC Voltage (V)"() -> (w198:T3)
                      n92 = local read "Second Harmonic"() -> (w188:bool)
                      n93 = call "DAQ_spectrum_analyzer_simultaneous_averaged_diag.vi"("Samples per Channel"="Samples per Channel", "minimum value"=w200, "DC voltage (V)"=w198, "maximum value"=w199, "LD channel"="LD Signal", "Error In"=w213, "Rate"="Rate", "Ref channel"="Reference Signal", "Second"=w188) -> ("Unbalanced?"=→"Signal Balance" →"Unbalanced?":bool, "raw signal waveform"=w204:waveform(dbl), "Calculated frequency"=w182:dbl, "Reference Timetrace"=w205:waveform(dbl), "1f 2f"=w203:T10, "error out"=w186:errorcluster)  [unwired: 5 out]
                      "2f Frequency (Hz)" <- w182
                      "1f 2f Spectral Peaks" <- w203
                      n94 = Build Array(w204, w205) -> (w206:waveform(dbl)[])
                      n95 = call <vilib>:"Application Directory.vi"() -> ("Application Directory"=w197:path)
                      n96 = local read "DC Voltage (V)"() -> (w183:T3)
                      n97 = local write "error out"(w186) -> ()
                      n98 = Path To String(path=w197) -> (string=w196:string)
                      n99 = Concatenate Strings(w196, "\\temp.txt" ("element")) -> (w194:string)
                      n100 = Unbundle(w203) -> ("1f Ampl (Vrms/Vdc)"=→"SA 1f (mv/V)":dbl, "2f Ampl (Vrms/Vdc)"=→"SA 2f (mv/V)":dbl)  [unwired: 2 out]
                      n101 = String To Path(string=w194) -> (path=w191:path)
                      "path" <- w191
                      n102 = Open/Create/Replace File(file path (use dialog)=w191, error in=w186, operation (0:open)=T7."replace or create") -> (refnum out=w190:refnum<file>, error out=w192:errorcluster)  [unwired: 3 in, 1 out]
                      n103 = Refnum to Path(1:w190) -> (0:w189:path)
                      n104 = call-poly <vilib>:"Export Waveforms to Spreadsheet File.vi"("header? (write header:T)"=FALSE, "append to file? (new file:F)"=TRUE ("header? (write header:T)"), "error in (no error)"=w192, "waveforms"=w206, "file path (dialog if empty)"=w189) -> ("error out"=w185:errorcluster)  [unwired: 5 in, 1 out]
                      n105 = case shown="True" "LockIn" {
                        tunnel: w186 -> [_ w240]
                        tunnel: w185 -> [w214 w235]
                        tunnel: [w214 w233] -> w184
                        tunnel: w183 -> [_ w228]
                        tunnel: w182 -> [_ w215]
                        frame False {
                        }
                        frame True {
                          w242 = 10178 items=["Finite Samples"=10178, "Continuous Samples"=10123] ("sample mode")
                          n106 = call "SR830_highfreq_readout.vi"("address string"="30", "X channel"=tag "Dev2/ai0", "number of samples per channel"=50000, "sample mode"=w242, "rate"=5000.0, "error in (no error)"=w240, "Y channel"=tag "Dev2/ai1", "Dc Voltage (V)"=w228) -> ("Lock In Signal Spectrum (mV/V) X,Y,R"=w217:cluster{"f0":dbl, "df":dbl, "magnitude":dbl[]}[], "Lockin R (mV/V)"=→"Lockin R":waveform(dbl), "Lock In Signal Spectrum (mV/V)"=w229:cluster{"f0":dbl, "df":dbl, "magnitude":dbl[]}, "Lockin X,Y,R (mV/V)"=→"Lockin X,Y,R":waveform(dbl)[], "Lockin Theta"=→"Lockin Theta":waveform(dbl), "error out"=w234:errorcluster)  [unwired: 2 out]
                          "PEM spectrum" <- w229
                          "PEM spectrum X,Y,R" <- w217
                          n107 = Merge Errors(w234, w235) -> (w233:errorcluster)
                          n108 = call "find_1f2f_diag.vi"("FFT - (RMS)"=w229, "Peak FWHM"=0.5, "Central Frequency"=w215) -> ("2f Peak Amplitude (mVrms/Vdc)"=→"2f PEM R":dbl, "1f Peak Amplitude(mVrms/Vdc)"=→"1f PEM R":dbl)  [unwired: 4 in, 3 out]
                          n109 = Index Array(array=w217, index=0) -> (element=w225:cluster{"f0":dbl, "df":dbl, "magnitude":dbl[]})
                          n110 = Index Array(array=w217, index=1) -> (element=w218:cluster{"f0":dbl, "df":dbl, "magnitude":dbl[]})
                          n111 = call "find_1f2f_diag.vi"("FFT - (RMS)"=w225, "Peak FWHM"=0.5, "Central Frequency"=w215) -> ("2f Peak Amplitude (mVrms/Vdc)"=→"2f PEM X":dbl, "1f Peak Amplitude(mVrms/Vdc)"=→"1f PEM X":dbl)  [unwired: 4 in, 3 out]
                          n112 = call "find_1f2f_diag.vi"("FFT - (RMS)"=w218, "Peak FWHM"=0.5, "Central Frequency"=w215) -> ("2f Peak Amplitude (mVrms/Vdc)"=→"2f PEM Y":dbl, "1f Peak Amplitude(mVrms/Vdc)"=→"1f PEM Y":dbl)  [unwired: 4 in, 3 out]
                        }
                      }
                    }
                  }
                  n113 = case shown="True" w144 {
                    tunnel: w147 -> [_ w156]
                    tunnel: w146 -> [_ w152]
                    frame False {
                    }
                    frame True {
                      n114 = for {
                        N: 10 -> [_]
                        tunnel: [w164] -> _ mode=indexing
                        tunnel: [w163] -> w160 mode=indexing
                        tunnel: [w162] -> _ mode=indexing
                        n115 = call "Lock_in_single_meas.vi"("Lock-in-Amplifier VISA"="Lock-in-Amplifier VISA") -> ("Lockin_phas"=w162:dbl, "Lockin_ampl"=w163:dbl, "Freq"=w164:dbl)  [unwired: 7 in, 1 out]
                        n116 = Wait (ms)(milliseconds to wait=u32 3000) -> ()  [unwired: 1 out]
                      }
                      n117 = call <vilib>:"Std Deviation and Variance.vi"("X"=w160) -> ("mean"=w159:dbl, "standard deviation"=w153:dbl)  [unwired: 1 in, 1 out]
                      n118 = Multiply(x=w159, y=1000.0) -> (x*y=w157:dbl)
                      n119 = Multiply(x=w153, y=1000.0) -> (x*y=w155:dbl)
                      n120 = Divide(x=w157, y=w156) -> (x/y=→"Lock_in (mV/V)":dbl)
                      n121 = Divide(x=w155, y=w152) -> (x/y=→"dLock_in (mV/V)":dbl)
                    }
                  }
                }
                frame "Process" {
                  n122 = Obtain Notifier(notification data type=FALSE) -> (notifier out=w261:refnum<notifier>, error out=w260:errorcluster)  [unwired: 3 in, 1 out]
                  n123 = stacked-sequence {
                    tunnel: w265 -> [w332 _]
                    tunnel: [w322 _] -> w269
                    tunnel: w261 -> [_ w385]
                    tunnel: [_ w383] -> w264
                    tunnel: w260 -> [_ w382]
                    tunnel: [_ w381] -> w262
                    frame #0 {
                      w321 = 1000
                      w306 = "Processing signal" ("Actual Task")
                      n124 = local write "Actual Task"(w306) -> ()
                      n125 = local read "Samples per Channel"() -> (w340:i32)
                      n126 = local read "Rate"() -> (w333:dbl)
                      n127 = local write "Quick Status 5"(w306) -> ()
                      n128 = local read "path"() -> (w308:path)
                      n129 = local read "DC Voltage (V)"() -> (w319:T3)
                      n130 = Multiply(x=1000.0, y="Stabilization Time (s)") -> (x*y=w311:dbl)
                      n131 = Wait (ms)(milliseconds to wait=w311) -> ()  [unwired: 1 out]
                      n132 = call "Lockin_Amplifier_diag_optional.vi"("Reference signal (dialog if empty)"=w308, "Sample Number"=w340, "DC(V)"=w319, "Cutoff Frequency"="Cutoff Frequency (Hz)", "dt"="dt (s)", "Window (s)"="Lock-in Time (s)", "Continous Lock-in"="Continous Lock-in", "Resolution"="Resolution (s)", "averaging time"="Averaging time (s)", "Error In"=w332, "Second"="Second Harmonic", "Sampling Freq"=w333, "tolerance (Deviation)"="Pike Removal (StDev)") -> ("Error Out"=w322:errorcluster, "Signal Spectrum"=w303:cluster{"f0":dbl, "df":dbl, "magnitude":dbl[]}[], "LockIN R (cont/disc)"=→"LockIN R (cont/disc)":waveform(dbl), "MLD & Phase"=w318:T11, "Time Domain Signal"=→"Time Domain Signal":cluster{"xi used":dbl[], "yi":dbl[]}[], "Timetrace_ref"=w305:waveform(dbl)[], "LockIN Theta (cont/disc)"=→"LockIN Theta (cont/disc)":waveform(dbl))  [unwired: 4 in, 4 out]
                      "Signal Spectrum (mVrms/Vdc)" <- w303
                      n133 = Unbundle(w318) -> ("MLD"=w317:dbl, "dMLD"=w316:dbl, "Phase"=→"Phase (deg)":dbl, "dPhase"=→"Phase  dev (deg)":dbl)
                      n134 = Index Array(array=w303, index=1) -> (element=→"Signal Spectrum (mVrms/Vdc) 2":cluster{"f0":dbl, "df":dbl, "magnitude":dbl[]})
                      n135 = local read "Dc mean"() -> (w320:dbl)
                      n136 = flat-sequence {
                        tunnel: w305 -> [w341]
                        tunnel: [w341] -> w304
                        frame #0 {
                          n137 = local write "Oscilloscope 2"(waveform(dbl)[] [{"t0"=timestamp(0 s since 1904-01-01), "dt"=0.001, "Y"=[]}, {"t0"=timestamp(0 s since 1904-01-01), "dt"=0.001, "Y"=[]}] ("Oscilloscope 2")) -> ()
                        }
                      }
                      n138 = Divide(x=w317, y=w320) -> (x/y=w331:dbl)
                      n139 = Divide(x=w316, y=w320) -> (x/y=w330:dbl)
                      n140 = local write "error out"(w322) -> ()
                      n141 = Multiply(x=w330, y=w321) -> (x*y=w327:dbl)
                      n142 = Multiply(x=w331, y=w321) -> (x*y=w328:dbl)
                      n143 = local read "Voltage Divider (10)"() -> (w329:bool)
                      n144 = case shown="False" w329 {
                        tunnel: w328 -> [w344 w349]
                        tunnel: w327 -> [w343 w348]
                        tunnel: [w344 w346] -> w325
                        tunnel: [w343 w345] -> w324
                        frame False {
                        }
                        frame True {
                          w347 = 10
                          n145 = Multiply(x=w349, y=w347) -> (x*y=w346:dbl)
                          n146 = Multiply(x=w348, y=w347) -> (x*y=w345:dbl)
                        }
                      }
                      "MLD (mV/V)" <- w325
                      "dMLD (mV/V)" <- w324
                      n147 = local write "Oscilloscope 2"(w304) -> ()
                    }
                    frame #1 {
                      w358 = "Plotting" ("Actual Task")
                      n148 = local read "Time Resolved"() -> (w367:bool)
                      n149 = case shown="True" w367 {
                        tunnel: [w397 w398] -> w366
                        frame False {
                          n150 = local read "2f Frequency (Hz)"() -> (w397:dbl)
                        }
                        frame True {
                          n151 = local read "Start time"() -> (w402:timestamp)
                          n152 = Get Date/Time In Seconds() -> (seconds since 1Jan1904=w403:timestamp)
                          n153 = Subtract(x=w403, y=w402) -> (x-y=w400:dbl)
                          n154 = To Double Precision Float(number=w400) -> (double precision float=w399:dbl)
                          n155 = Divide(x=w399, y=60.0) -> (x/y=w398:dbl)
                        }
                      }
                      n156 = local read "DC (V)"() -> (w373:cluster{dbl[], dbl[]})
                      n157 = local read "MLD Phase"() -> (w375:cluster{dbl[], dbl[]})
                      n158 = local read "DC Voltage (V) 2"() -> (w371:dbl)
                      n159 = Send Notification(notification=TRUE, notifier=w385, error in (no error)=w382) -> (notifier out=w383:refnum<notifier>, error out=w381:errorcluster)
                      n160 = Unbundle(w373) -> (w372:dbl[])  [unwired: 1 out]
                      n161 = Unbundle(w375) -> (w374:dbl[])  [unwired: 1 out]
                      n162 = local read "MLD (mV/V)"() -> (w380:dbl)
                      n163 = local read "dMLD (mV/V)"() -> (w379:dbl)
                      n164 = local read "Phase  dev (deg)"() -> (w378:dbl)
                      n165 = local read "LD array"() -> (w364:dbl[])
                      n166 = local read "Phase (deg)"() -> (w377:dbl)
                      n167 = Insert Into Array(array=w372, new element=w371) -> (w370:dbl[])  [unwired: 1 in]
                      n168 = local read "Frequency array"() -> (w365:dbl[])
                      n169 = local read "dPhase array"() -> (w388:dbl[])
                      n170 = local read "LD error array"() -> (w386:dbl[])
                      n171 = Insert Into Array(array=w365, new element=w366) -> (w369:dbl[])  [unwired: 1 in]
                      n172 = Insert Into Array(array=w386, new element=w379) -> (w363:dbl[])  [unwired: 1 in]
                      n173 = Insert Into Array(array=w374, new element=w378) -> (w389:dbl[])  [unwired: 1 in]
                      n174 = Insert Into Array(array=w388, new element=w377) -> (w391:dbl[])  [unwired: 1 in]
                      n175 = Insert Into Array(array=w364, new element=w380) -> (w350:dbl[])  [unwired: 1 in]
                      n176 = local write "Frequency array"(w369) -> ()
                      n177 = local write "LD array"(w350) -> ()
                      n178 = local write "Phase array"(w389) -> ()
                      n179 = local write "LD error array"(w363) -> ()
                      n180 = local read "SA 2f (mv/V)"() -> (w356:dbl)
                      n181 = Bundle("Frequency array"=w369, "LD array"=w350) -> (w387:T12)  [unwired: 1 in]
                      n182 = local write "dPhase array"(w391) -> ()
                      n183 = local read "2f Spectrum array"() -> (w354:dbl[])
                      n184 = call "XY error bars_diag.vi"("XY plot"=w387, "Yerror"=w363) -> ("Y error bars"=→"MLD Amplitude (mV/V)":cluster{dbl[], dbl[]})  [unwired: 6 in, 2 out]
                      n185 = Insert Into Array(array=w354, new element=w356) -> (w355:dbl[])  [unwired: 1 in]
                      "2f Spectrum array" <- w355
                      n186 = Array Size(array=w355) -> (size(s)=→"Measured Points":i32)
                      n187 = call <vilib>:"Std Deviation and Variance.vi"("X"=w355) -> ("mean"=w361:dbl, "standard deviation"=→"Delta":dbl)  [unwired: 1 in, 1 out]
                      "Detected Signal (mV/V)" <- w361
                      n188 = Bundle("Frequency array"=w369, w389) -> (w390:cluster{"Frequency array":dbl[], dbl[]})  [unwired: 1 in]
                      n189 = Bundle("Frequency array"=w369, w370) -> (→"DC (V)":cluster{"Frequency array":dbl[], dbl[]})  [unwired: 1 in]
                      n190 = call "XY error bars_diag.vi"("XY plot"=w390, "Yerror"=w391) -> ("Y error bars"=→"MLD Phase":cluster{dbl[], dbl[]})  [unwired: 6 in, 2 out]
                      n191 = local write "Actual Task"(w358) -> ()
                      n192 = local read "LD array"() -> (w353:dbl[])
                      n193 = local write "Quick Status 5"(w358) -> ()
                      n194 = Greater?(x=w361, y=2.0) -> (0:w362:bool)
                      n195 = case shown="True" w362 {
                        frame False {
                          n196 = local write "Quick Diagnosis"("Not infected" ("Quick Diagnosis")) -> ()
                          n197 = local write "Infected?"(FALSE ("Infected?")) -> ()
                        }
                        frame True {
                          "Infected?" <- TRUE ("Infected?")
                          "Quick Diagnosis" <- "Infected" ("Quick Diagnosis")
                        }
                      }
                      n198 = call <vilib>:"Std Deviation and Variance.vi"("X"=w353) -> ("mean"=→"mean MLD (mV/V)":dbl, "standard deviation"=→"Delta MLD":dbl)  [unwired: 1 in, 1 out]
                    }
                  }
                  n199 = while {
                    tunnel: w265 -> [w295]
                    tunnel: [w287] -> w268
                    tunnel: w261 -> [w294]
                    tunnel: w260 -> [w293]
                    tunnel: [w292] -> w259
                    stop <- w288 stop-if-true
                    n200 = Get Notifier Status(notifier=w294, error in (no error)=w293) -> (current notification=w289:bool, error out=w292:errorcluster)  [unwired: 3 out]
                    n201 = local read "DC Voltage (V) 2"() -> (w291:dbl)
                    n202 = local read "level B"() -> (w283:dbl)
                    n203 = local read "level A"() -> (w284:dbl)
                    n204 = local read "AC?"() -> (w275:bool)
                    n205 = local read "Reference Signal"() -> (w297:tag)
                    n206 = local read "V/div A"() -> (w286:dbl)
                    n207 = local read "LD Signal"() -> (w296:tag)
                    n208 = local read "V/div B"() -> (w285:dbl)
                    n209 = call "fast_scope_diag.vi"("Sensitivity"=T4."-10V..10V", "Reference Signal"=w297, "AC?"=w275, "mean"=w291, "LD Signal"=w296, "V/div"=w286, "error in (no error)"=w295, "Max frequency (Hz)"=200.0, "V/div in B"=w285, "level B"=w283, "Refresh in (s)"=1.0, "level A"=w284) -> ("levelA"=w281:dbl, "levelB"=w280:dbl, "Unbalanced"=w279:bool, "1f Peak (mv/V)"=w273:dbl, "MLD SA (mV/V)"=w272:dbl, "Scale Max"=w276:dbl, "Scale Min"=w278:dbl, "Frequency"=w274:dbl, "Spectrum"=w271:cluster{"f0":dbl, "df":dbl, "magnitude":dbl[]}, "V/div out"=w277:dbl, "Array"=w282:waveform(dbl)[], "error out"=w287:errorcluster)  [unwired: 4 in]
                    n210 = local write "1f SA (mV/V)"(w273) -> ()
                    n211 = local write "Spectrum (mVRMS/Vdc)"(w271) -> ()
                    n212 = local write "Oscilloscope"(w282) -> ()
                    n213 = local write "levelB"(w280) -> ()
                    n214 = local write "levelA"(w281) -> ()
                    n215 = local write "2f Frequency (Hz)"(w274) -> ()
                    n216 = property on="Oscilloscope" class="WFChart (strict)"("YScale.Increment"=w277, "YScale.Maximum"=w276, "YScale.Minimum"=w278) -> ()  [unwired: 2 in, 2 out]
                    n217 = local write "error out"(w287) -> ()
                    n218 = Not(x=w279) -> (.not. x?=w290:bool)
                    n219 = local write "Signal Balance"(w279) -> ()
                    n220 = And(x=w290, y=w289) -> (x .and. y?=w288:bool)
                    n221 = local write "MLD SA (mV/V)"(w272) -> ()
                  }
                  n222 = Merge Errors(w262, w259) -> (w263:errorcluster)
                  n223 = Release Notifier(notifier=w264, error in (no error)=w263) -> ()  [unwired: 1 in, 3 out]
                  n224 = Merge Errors(w269, w268) -> (w267:errorcluster)
                }
                frame "Save" {
                  n225 = local read "dLock_in (mV/V)"() -> (w417:dbl)
                  n226 = case shown="False" "Time Resolved" {
                    tunnel: [w470 w471] -> w411
                    frame False {
                      n227 = local read "2f Frequency (Hz)"() -> (w470:dbl)
                    }
                    frame True {
                      n228 = local read "Start time"() -> (w475:timestamp)
                      n229 = Get Date/Time In Seconds() -> (seconds since 1Jan1904=w476:timestamp)
                      n230 = Subtract(x=w476, y=w475) -> (x-y=w473:dbl)
                      n231 = To Double Precision Float(number=w473) -> (double precision float=w472:dbl)
                      n232 = Divide(x=w472, y=60.0) -> (x/y=w471:dbl)
                    }
                  }
                  n233 = local read "Lock_in (mV/V)"() -> (w418:dbl)
                  n234 = local read "SA 2f (mv/V)"() -> (w419:dbl)
                  n235 = local read "SA 1f (mv/V)"() -> (w420:dbl)
                  n236 = local read "Unbalanced?"() -> (w414:bool)
                  n237 = local read "Phase  dev (deg)"() -> (w427:dbl)
                  n238 = local read "Dc standard deviation"() -> (w425:dbl)
                  n239 = local read "dMLD (mV/V)"() -> (w421:dbl)
                  n240 = local read "MLD (mV/V)"() -> (w422:dbl)
                  n241 = local read "Phase (deg)"() -> (w428:dbl)
                  n242 = local read "Dc mean"() -> (w426:dbl)
                  n243 = Boolean To (0,1)(Boolean=w414) -> (0, 1=w416:i16)
                  n244 = To Double Precision Float(number=w416) -> (double precision float=w415:dbl)
                  n245 = local read "LockIn"() -> (w406:bool)
                  n246 = Build Array(w411, w422, w421, w420, w419, w418, w417, w428, w427, w426, w425, w415) -> (w405:dbl[])
                  n247 = case shown="False" w406 {
                    tunnel: w405 -> [w432 w440]
                    tunnel: [w432 w433] -> w404
                    frame False {
                    }
                    frame True {
                      n248 = local read "1f PEM R"() -> (w439:dbl)
                      n249 = local read "1f PEM X"() -> (w437:dbl)
                      n250 = local read "2f PEM R"() -> (w438:dbl)
                      n251 = local read "2f PEM X"() -> (w436:dbl)
                      n252 = local read "1f PEM Y"() -> (w435:dbl)
                      n253 = local read "2f PEM Y"() -> (w434:dbl)
                      n254 = Build Array (concatenate)(w440, w439, w438, w437, w436, w435, w434) -> (w433:dbl[])
                    }
                  }
                  n255 = Number To Decimal String(number=w411) -> (decimal integer string=w407:string)  [unwired: 1 in]
                  n256 = global read "Global 1_diag.vi" "Measurement File"() -> (w410:path)
                  n257 = Path To String(path=w410) -> (string=w408:string)
                  n258 = call-poly <vilib>:"Write To Spreadsheet File.vi"("format (%.3f)"="%g", "append to file? (new file:F)"=TRUE, "1D data"=w404, "file path (dialog if empty)"=w410) -> ()  [unwired: 4 in, 1 out]
                  n259 = Concatenate Strings(w408, w407) -> (w409:string)
                  n260 = case shown="True" "Save graphs" {
                    tunnel: w409 -> [_ w441]
                    frame False {
                    }
                    frame True {
                      n261 = Concatenate Strings(w441, "PEM_spectrum" ("element")) -> (w469:string)
                      n262 = Concatenate Strings(w441, "2f_spectrum" ("element")) -> (w448:string)
                      n263 = Concatenate Strings(w441, "PEM_Lockin_X_Y_R" ("element")) -> (w460:string)
                      n264 = Concatenate Strings(w441, "PEM_Lockin_theta" ("element")) -> (w459:string)
                      n265 = String To Path(string=w459) -> (path=w455:path)
                      n266 = String To Path(string=w469) -> (path=w462:path)
                      n267 = String To Path(string=w448) -> (path=w465:path)
                      n268 = String To Path(string=w460) -> (path=w452:path)
                      n269 = invoke on="Lockin X,Y,R" class="WFGraph (strict)" method="Export Image"("FileType"=enum32{"BMP", "EPS", "EMF", "PICT"}."BMP" ("File Type"), "Target"=enum32{"File", "Clipboard"}."File", "Path"=w452) -> ()  [unwired: 5 in, 8 out]
                      n270 = invoke on="PEM spectrum" class="WFGraph (strict)" method="Export Image"("FileType"=enum32{"BMP", "EPS", "EMF", "PICT"}."BMP" ("File Type"), "Target"=enum32{"File", "Clipboard"}."File", "Path"=w462) -> ()  [unwired: 5 in, 8 out]
                      n271 = invoke on="Signal Spectrum (mVrms/Vdc)" class="WFGraph (strict)" method="Export Image"("FileType"=enum32{"BMP", "EPS", "EMF", "PICT"}."BMP" ("File Type"), "Target"=enum32{"File", "Clipboard"}."File", "Path"=w465) -> ()  [unwired: 5 in, 8 out]
                      n272 = invoke on="Lockin Theta" class="WFGraph (strict)" method="Export Image"("FileType"=enum32{"BMP", "EPS", "EMF", "PICT"}."BMP" ("File Type"), "Target"=enum32{"File", "Clipboard"}."File", "Path"=w455) -> ()  [unwired: 5 in, 8 out]
                      n273 = local read "Lockin Theta"() -> (w445:waveform(dbl))
                      n274 = local read "Lockin X,Y,R"() -> (w446:waveform(dbl)[])
                      n275 = Concatenate Strings(w441, "PEM_Lockin_X,Y,R" ("element")) -> (w449:string)
                      n276 = Concatenate Strings(w441, "PEM_Lockin_Theta" ("element")) -> (w443:string)
                      n277 = String To Path(string=w449) -> (path=w447:path)
                      n278 = String To Path(string=w443) -> (path=w444:path)
                      n279 = call-poly <vilib>:"Export Waveforms to Spreadsheet File.vi"("waveforms"=w446, "file path (dialog if empty)"=w447) -> ()  [unwired: 8 in, 2 out]
                      n280 = call-poly <vilib>:"Export Waveforms to Spreadsheet File.vi"("waveform"=w445, "file path (dialog if empty)"=w444) -> ()  [unwired: 8 in, 2 out]
                    }
                  }
                  n281 = local read "Last Step?"() -> (w429:bool)
                  n282 = case shown="True" w429 {
                    tunnel: [State_machine_enum."Measure" State_machine_enum."Finished"] -> w430
                    frame False {
                    }
                    frame True {
                    }
                  }
                }
                frame "Finished" {
                  n283 = local read "Last Step?"() -> (w480:bool)
                }
              }
              n284 = local read "Stopped"() -> (w103:bool)
              n285 = Compound Arithmetic op=OR(w105, w104, w103) -> (w102:bool)
              "Actual State" <- w106
            }
          }
          frame #2 {
            # "Terminating"
            n286 = local read "Stopped"() -> (w483:bool)
            n287 = case shown="False" w483 {
              tunnel: w484 -> [w493 _]
              tunnel: [w492 w496] -> w481
              tunnel: w482 -> [w491 w496]
              frame False {
                w485 = "Measurement finished" ("Actual Task")
                n288 = local write "Reset?"(TRUE ("Reset?")) -> ()
                n289 = local write "Actual Task"(w485) -> ()
                n290 = local write "Quick Status 5"(w485) -> ()
                n291 = local read "Motor Voltage (V)"() -> (w486:dbl)
                n292 = local read "Motor Channel"() -> (w489:tag)
                n293 = call "gradual_motorset_diag.vi"("Initial Voltage (V)"=w486, "error in (no error)"=w491, "Steps"=500.0, "Next Voltage (V)"=0.0 ("Numeric"), "Physical Channel"=w489) -> ("error out"=w490:errorcluster)  [unwired: 6 in]
                n294 = Merge Errors(w493, w490) -> (w492:errorcluster)
              }
              frame True {
                n295 = local write "Stopped"(FALSE ("Stopped")) -> ()
              }
            }
            n296 = local write "error out"(w481) -> ()
          }
        }
      }
      frame "stop" {
        n297 = call <vilib>:"Three Button Dialog.vi"("Window Title (\"\")"="Stop Measurement" ("Window Title (\"\")"), "Right Button Text (\"Cancel\")"="Continue" ("Right Button Text (\"Cancel\")"), "Center Button Text (\"No\")"="Pause" ("Right Button Text (\"Cancel\")"), "Left Button Text (\"Yes\")"="Stop and Reset" ("Left Button Text (\"Yes\")"), "message"="Would You like to stop measurement?") -> ("Which Button?"=w500:T9)  [unwired: 6 in]
        n298 = case shown="\"Left Button\", Default" w500 {
          tunnel: w499 -> [w508 w528 w560]
          tunnel: [w507 w527 w560] -> w498
          tunnel: w497 -> [_ w526 w559]
          frame "Left Button", Default {
            # "Stop and reset"
            n299 = local write "Reset?"(TRUE ("Reset?")) -> ()
            n300 = local read "Motor Channel"() -> (w509:tag)
            n301 = global read "Global 1_diag.vi" "Measurement File"() -> (w511:path)
            n302 = call "motor_control_voltage.vi"("Error In"=w508, "Numeric"=0.0, "Physical Channel"=w509) -> ("error out"=w507:errorcluster)  [unwired: 8 in]
            n303 = Not A Number/Path/Refnum?(number/path/refnum=w511) -> (NaN/Path/Refnum?=w512:bool)
            n304 = Empty String/Path?(string/path=w511) -> (empty?=w513:bool)
            n305 = Or(x=w512, y=w513) -> (x .or. y?=w514:bool)
            n306 = case shown="False" w514 {
              tunnel: w511 -> [w515 _]
              frame False {
                n307 = local read "Phase  dev (deg)"() -> (w518:dbl)
                n308 = local read "Dc standard deviation"() -> (w516:dbl)
                n309 = local read "2f Frequency (Hz)"() -> (w522:dbl)
                n310 = local read "dMLD (mV/V)"() -> (w520:dbl)
                n311 = local read "MLD (mV/V)"() -> (w521:dbl)
                n312 = local read "Phase (deg)"() -> (w519:dbl)
                n313 = local read "Dc mean"() -> (w517:dbl)
                n314 = Build Array(w522, w521, w520, w519, w518, w517, w516) -> (w525:dbl[])
                n315 = call-poly <vilib>:"Write To Spreadsheet File.vi"("format (%.3f)"="%g", "append to file? (new file:F)"=TRUE, "1D data"=w525, "file path (dialog if empty)"=w515) -> ()  [unwired: 4 in, 1 out]
              }
              frame True {
              }
            }
          }
          frame "Center Button" {
            # "Pause"
            n316 = local write "Reset?"(FALSE ("Reset?")) -> ()
            n317 = local write "Stopped"(FALSE ("Stopped")) -> ()
            n318 = local write "Actual Task"("Paused" ("Actual Task")) -> ()
            n319 = while {
              tunnel: w528 -> [w550]
              tunnel: [w549] -> w527
              tunnel: w526 -> [w546]
              stop <- w547 stop-if-true
              n320 = local read "Reference Signal"() -> (w554:tag)
              n321 = local read "LD Signal"() -> (w555:tag)
              n322 = Get Queue Status(queue=w546) -> (# elements in queue=w548:i32)  [unwired: 2 in, 7 out]
              n323 = local read "DC Voltage (V) 2"() -> (w545:dbl)
              n324 = local read "AC?"() -> (w544:bool)
              n325 = Greater Than 0?(x=w548) -> (x > 0?=w547:bool)
              n326 = local read "V/div B"() -> (w542:dbl)
              n327 = local read "level A"() -> (w541:dbl)
              n328 = local read "level B"() -> (w540:dbl)
              n329 = local read "V/div A"() -> (w543:dbl)
              n330 = call "fast_scope_diag.vi"("Sensitivity"=T4."-10V..10V", "Reference Signal"=w554, "AC?"=w544, "mean"=w545, "LD Signal"=w555, "V/div"=w543, "error in (no error)"=w550, "Max frequency (Hz)"=200.0, "V/div in B"=w542, "level B"=w540, "Refresh in (s)"=1.0, "level A"=w541) -> ("levelA"=w539:dbl, "levelB"=w538:dbl, "Unbalanced"=w533:bool, "Scale Max"=w536:dbl, "Scale Min"=w535:dbl, "Spectrum"=w532:cluster{"f0":dbl, "df":dbl, "magnitude":dbl[]}, "V/div out"=w534:dbl, "Array"=w537:waveform(dbl)[], "error out"=w549:errorcluster)  [unwired: 4 in, 3 out]
              n331 = local write "levelA"(w539) -> ()
              n332 = local write "levelB"(w538) -> ()
              n333 = local write "Signal Spectrum (mVrms/Vdc) 2"(w532) -> ()
              n334 = local write "Spectrum (mVRMS/Vdc)"(w532) -> ()
              n335 = local write "Signal Balance"(w533) -> ()
              n336 = local write "Oscilloscope"(w537) -> ()
              n337 = property on="Oscilloscope" class="WFChart (strict)"("YScale.Increment"=w534, "YScale.Maximum"=w536, "YScale.Minimum"=w535) -> ()  [unwired: 2 in, 2 out]
            }
          }
          frame "Right Button" {
            # "Continue"
            n338 = Enqueue Element(queue=w559, element=User_buttons_enum."start") -> ()  [unwired: 2 in, 3 out]
            n339 = local write "Stopped"(FALSE ("Stopped")) -> ()
            "Reset?" <- FALSE ("Reset?")
          }
        }
      }
      frame "exit" {
        # "This will stop the consumer loop, thus exit this\nportion of the program."
      }
      frame "New" {
        n340 = call "Create_file_diag.vi"("error in (no error)"=w565) -> ("error out"=w564:errorcluster, "Measurement File out"=w563:path)  [unwired: 9 in]
        n341 = local write "Measurement File"(w563) -> ()
      }
      frame "Scope" {
        w566 = 10106 items=["default"=-1, "RSE"=10083, "NRSE"=10078, "Differential"=10106, "Pseudodifferential"=12529] ("input terminal configuration")
        w591 = 10123 items=["Finite Samples"=10178, "Continuous Samples"=10123, "Hardware Timed Single Point"=12522]  # sample mode
        w598 = FALSE  # auto cleanup
        n342 = Divide(x=1.0, y="rate") -> (x/y=→"dt":dbl)
        n343 = local read "DC Voltage DAQ"() -> (w568:tag)
        n344 = call <vilib>:"DAQmx Create Task.vi"("auto cleanup"=w598, "error in"=w575) -> ("task out"=w574:refnum<k21>, "error out"=w573:errorcluster)  [unwired: 12 in]
        n345 = local read "Reference Signal"() -> (w600:tag)
        n346 = call-poly <vilib>:"DAQmx Create Virtual Channel.vi"("task in"=w574, "maximum value"=10.0, "minimum value"=-10.0, "input terminal configuration"=w566, "physical channels"=w568, "error in"=w573) -> ("task out"=w572:refnum<k21>, "error out"=w571:errorcluster)  [unwired: 8 in]
        n347 = call-poly <vilib>:"DAQmx Create Virtual Channel.vi"("task in"=w572, "maximum value"=10.0, "minimum value"=-10.0, "input terminal configuration"=w566, "physical channels"=w600, "error in"=w571) -> ("task out"=w594:refnum<k21>, "error out"=w595:errorcluster)  [unwired: 8 in]
        n348 = local read "LD Signal"() -> (w599:tag)
        n349 = case shown="\"-1V..1V\", Default" "Sensitivity" {
          tunnel: [-1.0 ("maximum value") -1.25 ("maximum value") -2.0 ("maximum value") -2.5 ("maximum value") -4.0 ("maximum value") -5.0 ("maximum value") -10.0 ("maximum value")] -> w589
          tunnel: [1.0 ("maximum value") 1.25 ("maximum value") 2.0 ("maximum value") 2.5 ("maximum value") 4.0 ("maximum value") 5.0 ("maximum value") 10.0 ("maximum value")] -> w588
          frame "-1V..1V", Default {
          }
          frame "-1.25V..1.25V" {
          }
          frame "-2V..2V" {
          }
          frame "-2.5V..2.5V" {
          }
          frame "-4V..4V" {
          }
          frame "-5V..5V" {
          }
          frame "-10V..10V" {
          }
        }
        n350 = call-poly <vilib>:"DAQmx Create Virtual Channel.vi"("task in"=w594, "maximum value"=w588, "minimum value"=w589, "input terminal configuration"=w566, "physical channels"=w599, "error in"=w595) -> ("task out"=w592:refnum<k21>, "error out"=w593:errorcluster)  [unwired: 8 in]
        n351 = call-poly <vilib>:"DAQmx Timing.vi"("task/channels in"=w592, "sample mode"=w591, "samples per channel"="samples per channel", "rate"="rate", "error in"=w593) -> ("task out"=w579:refnum<k21>, "error out"=w577:errorcluster)  [unwired: 9 in]
        n352 = property class="DAQmx Channel"(reference=w579, error in=w577, "AI.UsbXferReqCount"=u32 1) -> (reference out=w578:refnum<k21>, error out=w576:errorcluster)
        n353 = while {
          tunnel: [w636] -> w582
          tunnel: w576 -> [w621]
          tunnel: w578 -> [w626]
          tunnel: "samples per channel" -> [w625]
          tunnel: [w623] -> w583
          tunnel: w567 -> [w615]
          stop <- w637 stop-if-true
          n354 = Obtain Queue(element data type=dbl[][] [] ("data")) -> (queue out=w641:refnum<queue>)  [unwired: 4 in, 2 out]
          n355 = while {
            tunnel: w641 -> [w651]
            shift-right: [w645] -> w620
            shift-left: dbl[][] [] ("element data type") -> [w652]
            tunnel: w615 -> [w643]
            i -> [w648]
            stop <- w644 stop-if-true
            n356 = Equal?(x=0, y=w648) -> (x = y?=w646:bool)
            n357 = Dequeue Element(queue=w651) -> (element=w650:dbl[][], error out=w649:errorcluster)  [unwired: 2 in, 2 out]
            n358 = case shown="No Error" w649 {
              tunnel: w650 -> [w664 _]
              tunnel: w652 -> [w685 w768]
              tunnel: w646 -> [w684 _]
              tunnel: [w673 w768] -> w645
              tunnel: [FALSE TRUE] -> w644
              tunnel: w643 -> [w654 _]
              frame No Error {
                n359 = local read "Second Harmonic"() -> (w661:bool)
                n360 = Transpose 2D Array(2D array=w664) -> (transposed array=w663:dbl[][])
                n361 = Index Array(array=w663, index (col)=2) -> (element=w662:dbl[])  [unwired: 1 in]
                n362 = Index Array(array=w663, index (col)=1) -> (element=w668:dbl[])  [unwired: 1 in]
                n363 = Build Array(w668, w662) -> (w666:dbl[][])
                n364 = Transpose 2D Array(2D array=w666) -> (transposed array=w665:dbl[][])
                n365 = Insert Into Array(array=w685, new element=w665) -> (w667:dbl[][])  [unwired: 2 in]
                n366 = local read "dt"() -> (w678:dbl)
                n367 = call "Scopeset_diag.vi"("Ref_MLD measurement"=w665, "V/div in B"="V/div B", "Second"=w661, "AC?"="AC?", "V/div in A"="V/div A", "level B"="level B", "level A"="level A", "dt"=w678) -> ("UP"=w659:bool, "Down"=w660:bool, "V/div out"=w692:dbl, "Ref_MLD_triggered"=w686:dbl[][], "levelB"=→"levelB":dbl, "MLD_mean"=w658:dbl, "Scale Max"=w694:dbl, "Scale Min"=w693:dbl, "levelA"=→"levelA":dbl, "Array"=w653:waveform(dbl)[], "Frequency"=w675:dbl)  [unwired: 7 in, 2 out]
                "Oscilloscope" <- w653
                "Up" <- w659
                "Down" <- w660
                "Oscilloscope 2" <- w653
                n368 = property on="Oscilloscope" class="WFChart (strict)"("YScale.Increment"=w692, "YScale.Maximum"=w694, "YScale.Minimum"=w693) -> ()  [unwired: 2 in, 2 out]
                n369 = local write "2f Frequency (Hz)"(w675) -> ()
                n370 = local write "2f Frequency (Hz)"(w675) -> ()
                n371 = case shown="False" w684 {
                  tunnel: w686 -> [_ w766]
                  tunnel: w667 -> [w765 _]
                  tunnel: [w765 w766] -> w673
                  frame False {
                  }
                  frame True {
                  }
                }
                n372 = Index Array(array=w663, index (col)=0) -> (element=w672:dbl[])  [unwired: 1 in]
                n373 = call-poly <vilib>:"Mean.vi"("X"=w672) -> ("mean"=w656:dbl)  [unwired: 1 out]
                "DC Voltage (V)" <- w656
                n374 = local write "DC Voltage (V) 2"(w656) -> ()
                n375 = Index Array(array=w673, index (col)=1 ("disabled index (col)")) -> (element=w655:dbl[])  [unwired: 1 in]
                n376 = case shown="True" "QuickDiag" {
                  tunnel: w660 -> [_ w702]
                  tunnel: w659 -> [_ w701]
                  tunnel: w658 -> [_ w700]
                  tunnel: w656 -> [_ w699]
                  tunnel: w655 -> [_ w698]
                  tunnel: w653 -> [_ _]
                  tunnel: w654 -> [_ w697]
                  frame False {
                  }
                  frame True {
                    n377 = stacked-sequence {
                      tunnel: w702 -> [_ _ w726 _]
                      tunnel: w701 -> [_ _ w725 _]
                      tunnel: w700 -> [_ _ w722 _]
                      tunnel: w699 -> [w706 w716 _ _]
                      tunnel: w698 -> [_ w715 _ _]
                      tunnel: w697 -> [_ _ _ _]
                      frame #0 {
                        n378 = local write "Quick Status 5"("Checking LASER" ("Quick Status 5")) -> ()
                        n379 = Greater?(x=w706, y=1.0) -> (0:w703:bool)
                        n380 = case shown="True" w703 {
                          frame False {
                            n381 = local write "Laser Intensity"("Laser Intensity: Too low" ("Laser Intensity")) -> ()
                            n382 = local write "Laser Intensity"(FALSE ("Laser Intensity")) -> ()
                          }
                          frame True {
                            "Laser Intensity" <- TRUE ("Laser Intensity")
                            "Laser Intensity" <- "Laser Intensity: OK" ("Laser Intensity")
                          }
                        }
                      }
                      frame #1 {
                        n383 = call <vilib>:"Std Deviation and Variance.vi"("X"=w715) -> ("standard deviation"=w714:dbl)  [unwired: 1 in, 2 out]
                        n384 = Divide(x=w714, y=w716) -> (x/y=w713:dbl)
                        "x/y" <- w713
                        n385 = Less?(x=w713, y=0.05) -> (x < y?=w711:bool)
                        n386 = case shown="True" w711 {
                          frame False {
                            n387 = local write "Laser Noise"("Laser Noise: Too High" ("Laser Noise")) -> ()
                            n388 = local write "Laser Noise"(FALSE ("Laser Noise")) -> ()
                          }
                          frame True {
                            "Laser Noise" <- TRUE ("Laser Noise")
                            "Laser Noise" <- "Laser Noise: OK" ("Laser Noise")
                          }
                        }
                      }
                      frame #2 {
                        n389 = Absolute Value(x=w722) -> (abs(x)=w724:dbl)
                        n390 = Less?(x=w724, y=0.2) -> (x < y?=w721:bool)
                        n391 = case shown="True" w721 {
                          frame False {
                            n392 = local write "Signal Balance"(FALSE ("Signal Balance")) -> ()
                            "Signal Balance" <- "Signal Balance : Unbalanced" ("Signal Balance")
                          }
                          frame True {
                            n393 = local write "Signal Balance"("Signal Balance: OK" ("Signal Balance")) -> ()
                            "Signal Balance" <- TRUE ("Signal Balance")
                          }
                        }
                        "Down 2" <- w726
                        "Up 2" <- w725
                      }
                      frame #3 {
                        n394 = local read "Laser Intensity"() -> (w732:bool)
                        n395 = local read "Laser Noise"() -> (w733:bool)
                        n396 = local read "Signal Balance"() -> (w734:bool)
                        n397 = Compound Arithmetic op=AND(w732, w733, w734) -> (w731:bool)
                        n398 = case shown="True" w731 {
                          frame False {
                          }
                          frame True {
                            n399 = stacked-sequence {
                              frame #0 {
                                n400 = property on="Constant Motor Voltage" class="DigNum (strict)"("Val(Sgnl)"=1.0 ("Value (Signaling)")) -> ()  [unwired: 2 in, 2 out]
                                n401 = local write "Quick Status 5"("LASER OK, Motor ON" ("Quick Status 5")) -> ()
                              }
                              frame #1 {
                                n402 = local read "2f Frequency (Hz)"() -> (w741:T3)
                                n403 = Greater?(x=w741, y=T3 18.0) -> (0:w738:bool)
                                n404 = Less?(x=w741, y=T3 21.0) -> (x < y?=w737:bool)
                                n405 = And(x=w738, y=w737) -> (x .and. y?=w739:bool)
                                n406 = case shown="True" w739 {
                                frame False {
                                n407 = local write "Motor"("Motor:...  " ("Motor")) -> ()
                                n408 = local write "Motor"(FALSE ("Motor")) -> ()
                                }
                                frame True {
                                n409 = local write "QuickDiag"(FALSE ("QuickDiag")) -> ()
                                n410 = local write "Ready?"(TRUE ("Ready?")) -> ()
                                n411 = property on="Measure" class="Bool"("DisabledEnum"=T8."Enabled" ("Disabled")) -> ()  [unwired: 2 in, 2 out]
                                "Motor" <- TRUE ("Motor")
                                "Motor" <- "Motor: OK" ("Motor")
                                }
                                }
                              }
                            }
                          }
                        }
                      }
                    }
                  }
                }
                n412 = Bundle By Name("Y"=w655, "dt"=w678) -> (w671:waveform(dbl))  [unwired: 1 in]
                n413 = case shown="False" "Lock In" {
                  tunnel: w656 -> [_ w750]
                  frame False {
                  }
                  frame True {
                    n414 = local read "Lock-in-Amplifier VISA"() -> (w754:refnum<visa-resource-name>)
                    n415 = call "Lock_in_single_meas.vi"("Lock-in-Amplifier VISA"=w754) -> ("Lockin_ampl"=w752:dbl, "Freq"=→"Lockin_freq":dbl)  [unwired: 7 in, 2 out]
                    n416 = xnode "LIA calc"("X1"=w752, "X2"=w750) -> ("Result"=→"MLD LIA (mV/V)":dbl)  [unwired: 1 in, 1 out]
                  }
                }
                n417 = call "Fast_spectrum_analyzer_diag.vi"("mean"=w656, "Waveform"=w671, "Frequency"=w675) -> ("error out"=w683:errorcluster, "MLD SA (mV/V)"=w677:dbl, "Spectrum (mV/V)"=→"Spectrum (mVRMS/Vdc)":cluster{"f0":dbl, "df":dbl, "magnitude":dbl[]}, "1f Peak (mv/V)"=w676:dbl)  [unwired: 5 in]
                n418 = local write "MLD SA (mV/V)"(w677) -> ()
                n419 = local write "1f SA (mV/V)"(w676) -> ()
                n420 = local write "error out"(w683) -> ()
              }
              frame Error {
              }
            }
          }
          n421 = while {
            tunnel: [w784] -> w623
            shift-right: [w769] -> w624
            shift-left: w621 -> [w785]
            tunnel: [w781] -> _
            tunnel: w641 -> [w780]
            tunnel: [w778] -> w640
            tunnel: w626 -> [w777]
            tunnel: w625 -> [w776]
            tunnel: ["stop"] -> w616
            i -> [w775]
            stop <- w781 stop-if-true
            w782 = 10.0  # timeout (s)
            n422 = Subtract(x="Refresh in (s)", y=i8 2) -> (x-y=w773:i8)
            n423 = Less?(x=w773, y=w775) -> (x < y?=w774:bool)
            n424 = call-poly <vilib>:"DAQmx Read.vi"("task/channels in"=w777, "number of samples per channel"=w776, "timeout"=w782, "error in"=w785) -> ("task out"=w784:refnum<k21>, "data"=w779:dbl[][], "error out"=w769:errorcluster)  [unwired: 9 in]
            n425 = Unbundle By Name(w769) -> ("status"=w783:bool)
            n426 = local write "error out"(w769) -> ()
            n427 = Enqueue Element(queue=w780, element=w779) -> (queue out=w778:refnum<queue>)  [unwired: 2 in, 2 out]
            n428 = Compound Arithmetic op=OR(w783, "stop", w774) -> (w781:bool)
            "result" <- w781
          }
          n429 = local read "Continous Lock-in"() -> (w617:bool)
          n430 = Merge Errors(w624) -> (w635:errorcluster)
          n431 = case shown="True" w616 {
            frame False {
            }
            frame True {
              n432 = local write "stop"(FALSE ("stop")) -> ()
            }
          }
          n433 = Release Queue(queue=w640, error in (no error)=w635) -> (error out=w636:errorcluster)  [unwired: 1 in, 2 out]
          n434 = local read "DC Voltage (V) 2"() -> (w618:dbl)
          n435 = local read "Refresh in (s)"() -> (w631:i8)
          n436 = Array Size(array=w620) -> (size(s)=w629:i32[])
          n437 = Transpose 2D Array(2D array=w620) -> (transposed array=w619:dbl[][])
          n438 = Index Array(array=w629, index=0) -> (element=w630:i32)
          n439 = local read "rate"() -> (w633:dbl)
          n440 = local read "dt"() -> (w634:dbl)
          n441 = local read "Second Harmonic"() -> (w628:bool)
          n442 = call "Lockin_Amplifier_diag_fast.vi"("Refresh in (s)"=w631, "dt"=w634, "mean"=w618, "Continous Lock-in"=w617, "Ref_MLD measurement"=w619, "Second"=w628, "Number of samples"=w630, "Sampling frequency"=w633) -> ("Result 2"=w622:dbl, "Result"=→"dLD_RMS":dbl)  [unwired: 6 in]
          n443 = local write "MLD Sim. LIA (mV/V)"(w622) -> ()
          n444 = Compound Arithmetic op=OR(w616, w636) -> (w637:bool)
        }
        n445 = call <vilib>:"DAQmx Clear Task.vi"("task in"=w583, "error in"=w582) -> ("error out"=w581:errorcluster)  [unwired: 13 in]
      }
    }
    n446 = Unbundle By Name(w14) -> ("status"=w13:bool)
    n447 = Or(x=w13, y=w12) -> (x .or. y?=w11:bool)
  }
  n448 = while {
    shift-right: [w788] -> w6
    shift-left: w9 -> [w791]
    tunnel: w3 -> [w792]
    tunnel: [w786] -> w7
    stop <- w789 stop-if-true
    # "This loop is the producer loop."
    n449 = event shown="[5] \"Start Scope\": Value Change" {
      selector: _ -> [_ _ _ _ _ _ _ _ _ _ _ _ _ _]
      dyn-events: _ -> [_ _ _ _ _ _ _ _ _ _ _ _ _ _]
      timeout: _ -> [_ _ _ w811 _ _ _ _ _ _ _ _ _ _]
      tunnel: w792 -> [w797 w802 w809 w813 w822 w828 _ _ _ _ _ _ _ w904]
      tunnel: w791 -> [w796 w803 w807 w816 w821 w827 w834 _ _ _ _ _ w897 w903]
      tunnel: [w795 w800 w806 w815 w819 w825 w831 _ _ _ _ _ w897 w902] -> w788
      tunnel: [_ _ _ "EXIT" _ _ _ _ _ _ _ _ _ _] -> w790
      tunnel: [w794 w801 w808 w814 w820 w826 _ _ _ _ _ _ _ w901] -> w786
      tunnel: [_ _ _ w811 _ _ _ _ _ _ _ _ _ _] -> _
      event "Start Measurement Button": Value Change {
        n450 = event-data() -> ()  [unwired: 1 in, 1 out]
        n451 = Enqueue Element(queue=w797, element=User_buttons_enum."start", error in (no error)=w796) -> (queue out=w794:refnum<queue>, error out=w795:errorcluster)  [unwired: 1 in, 1 out]
      }
      event "Stop Measurement": Value Change {
        n452 = event-data() -> ()  [unwired: 1 in, 1 out]
        n453 = Enqueue Element(queue=w802, element=User_buttons_enum."stop", error in (no error)=w803) -> (queue out=w801:refnum<queue>, error out=w800:errorcluster)  [unwired: 1 in, 1 out]
        "Stopped" <- TRUE
      }
      event "Measure": Value Change {
        n454 = event-data() -> ()  [unwired: 1 in, 3 out]
        n455 = local write "stop"(TRUE ("stop")) -> ()
        n456 = local write "QuickDiag"(FALSE ("QuickDiag")) -> ()
        n457 = Enqueue Element(queue=w809, element=User_buttons_enum."start", error in (no error)=w807) -> (queue out=w808:refnum<queue>, error out=w806:errorcluster)  [unwired: 1 in, 1 out]
      }
      event "EXIT": Value Change {
        n458 = event-data() -> ()  [unwired: 1 in, 1 out]
        n459 = Enqueue Element(queue=w813, element=User_buttons_enum."exit", error in (no error)=w816) -> (queue out=w814:refnum<queue>, error out=w815:errorcluster)  [unwired: 1 in, 1 out]
      }
      event "New File": Value Change {
        n460 = event-data() -> ()  [unwired: 1 in, 1 out]
        n461 = Enqueue Element(queue=w822, element=User_buttons_enum."New", error in (no error)=w821) -> (queue out=w820:refnum<queue>, error out=w819:errorcluster)  [unwired: 1 in, 1 out]
      }
      event "Start Scope": Value Change {
        n462 = event-data() -> ()  [unwired: 1 in, 1 out]
        n463 = Enqueue Element(queue=w828, element=User_buttons_enum."Scope", error in (no error)=w827) -> (queue out=w826:refnum<queue>, error out=w825:errorcluster)  [unwired: 1 in, 1 out]
        n464 = local write "QuickDiag"(FALSE ("QuickDiag")) -> ()
      }
      event "Constant Motor Voltage": Value Change {
        n465 = event-data() -> ()  [unwired: 1 in, 1 out]
        n466 = local read "Motor Voltage (V)"() -> (w833:dbl)
        n467 = local read "Motor Channel"() -> (w836:tag)
        n468 = call "gradual_motorset_diag.vi"("Initial Voltage (V)"=w833, "error in (no error)"=w834, "Steps"=100.0, "Next Voltage (V)"="Constant Motor Voltage", "Physical Channel"=w836) -> ("error out"=w832:errorcluster)  [unwired: 6 in]
        n469 = case shown="Error" w832 {
          selector: w832 -> [w838 w839]
          tunnel: [w838 w839] -> w831
          tunnel: "Constant Motor Voltage" -> [w837 _]
          tunnel: [w837 0.0 ("Constant Motor Voltage")] -> w829
          frame No Error {
          }
          frame Error {
          }
        }
        n470 = local write "Motor Voltage (V)"(w829) -> ()
      }
      event "Convert dT": Value Change {
        n471 = event-data() -> ()  [unwired: 1 in, 1 out]
        n472 = local read "dT/T (%)"() -> (w849:dbl)
        n473 = local read "Dilution"() -> (w843:dbl)
        n474 = Multiply(x=w849, y=1200.0) -> (x*y=w850:dbl)
        n475 = Divide(x=w849, y=0.0012) -> (x/y=w842:dbl)
        n476 = Multiply(x=w843, y=w842) -> (x*y=w841:dbl)
        n477 = local write "Undiluted cc.\n (ng/ml)"(w841) -> ()
        n478 = local write "MLD (mV/V)"(w850) -> ()
        n479 = Multiply(x=w841, y=2.0) -> (x*y=w846:dbl)
        n480 = Multiply(x=w846, y=2e-05) -> (x*y=w844:dbl)
        n481 = local write "Undiluted \nParasitemia (%)"(w844) -> ()
        n482 = local write "Parasites/ul\nof Blood"(w846) -> ()
      }
      event "Convert mld": Value Change {
        n483 = event-data() -> ()  [unwired: 1 in, 1 out]
        n484 = local read "MLD (mV/V)"() -> (w854:dbl)
        n485 = local read "Dilution"() -> (w856:dbl)
        n486 = Divide(x=w854, y=1200.0) -> (x/y=w853:dbl)
        n487 = Divide(x=w853, y=0.0012) -> (x/y=w855:dbl)
        n488 = Multiply(x=w856, y=w855) -> (x*y=w852:dbl)
        n489 = local write "Undiluted cc.\n (ng/ml)"(w852) -> ()
        n490 = local write "dT/T (%)"(w853) -> ()
        n491 = Multiply(x=w852, y=2.0) -> (x*y=w859:dbl)
        n492 = Multiply(x=w859, y=2e-05) -> (x*y=w857:dbl)
        n493 = local write "Undiluted \nParasitemia (%)"(w857) -> ()
        n494 = local write "Parasites/ul\nof Blood"(w859) -> ()
      }
      event "Convert cc": Value Change {
        n495 = event-data() -> ()  [unwired: 1 in, 1 out]
        n496 = local read "Undiluted cc.\n (ng/ml)"() -> (w863:dbl)
        n497 = local read "Dilution"() -> (w869:dbl)
        n498 = Divide(x=w863, y=w869) -> (x/y=w868:dbl)
        n499 = Multiply(x=w863, y=2.0) -> (x*y=w870:dbl)
        n500 = Multiply(x=0.0012 ("y"), y=w868) -> (x*y=w866:dbl)
        n501 = local write "Parasites/ul\nof Blood"(w870) -> ()
        n502 = local write "dT/T (%)"(w866) -> ()
        n503 = Multiply(x=w870, y=2e-05) -> (x*y=w873:dbl)
        n504 = local write "Undiluted \nParasitemia (%)"(w873) -> ()
        n505 = Multiply(x=1200.0 ("y"), y=w866) -> (x*y=w864:dbl)
        n506 = local write "MLD (mV/V)"(w864) -> ()
      }
      event "Convert parasitemia": Value Change {
        n507 = event-data() -> ()  [unwired: 1 in, 1 out]
        n508 = local read "Undiluted \nParasitemia (%)"() -> (w880:dbl)
        n509 = Divide(x=w880, y=2e-05) -> (x/y=w883:dbl)
        n510 = local read "Dilution"() -> (w884:dbl)
        n511 = Divide(x=w883, y=2.0) -> (x/y=w875:dbl)
        n512 = Divide(x=w875, y=w884) -> (x/y=w874:dbl)
        n513 = Multiply(x=0.0012 ("y"), y=w874) -> (x*y=w878:dbl)
        n514 = local write "dT/T (%)"(w878) -> ()
        n515 = local write "Undiluted cc.\n (ng/ml)"(w875) -> ()
        n516 = local write "Parasites/ul\nof Blood"(w883) -> ()
        n517 = Multiply(x=1200.0 ("y"), y=w878) -> (x*y=w876:dbl)
        n518 = local write "MLD (mV/V)"(w876) -> ()
      }
      event "Convert parasiteno": Value Change {
        n519 = event-data() -> ()  [unwired: 1 in, 1 out]
        n520 = local read "Parasites/ul\nof Blood"() -> (w887:dbl)
        n521 = Multiply(x=w887, y=2e-05) -> (x*y=w895:dbl)
        n522 = local read "Dilution"() -> (w894:dbl)
        n523 = Divide(x=w887, y=2.0) -> (x/y=w886:dbl)
        n524 = local write "Undiluted \nParasitemia (%)"(w895) -> ()
        n525 = Divide(x=w886, y=w894) -> (x/y=w885:dbl)
        n526 = Multiply(x=0.0012 ("y"), y=w885) -> (x*y=w890:dbl)
        n527 = local write "dT/T (%)"(w890) -> ()
        n528 = local write "Undiluted cc.\n (ng/ml)"(w886) -> ()
        n529 = Multiply(x=1200.0 ("y"), y=w890) -> (x*y=w888:dbl)
        n530 = local write "MLD (mV/V)"(w888) -> ()
      }
      event "Timer Start": Value Change {
        n531 = event-data() -> ()  [unwired: 1 in, 3 out]
        n532 = Get Date/Time In Seconds() -> (seconds since 1Jan1904=w896:timestamp)
        n533 = local write "Start time"(w896) -> ()
      }
      event "Run Quick Diagnostics": Value Change {
        n534 = event-data() -> ()  [unwired: 1 in, 3 out]
        n535 = local write "QuickDiag"(TRUE ("QuickDiag")) -> ()
        n536 = Enqueue Element(queue=w904, element=User_buttons_enum."Scope", error in (no error)=w903) -> (queue out=w901:refnum<queue>, error out=w902:errorcluster)  [unwired: 1 in, 1 out]
        n537 = property on="Measure" class="Bool"("DisabledEnum"=T8."Disabled and Grayed Out" ("Disabled")) -> ()  [unwired: 2 in, 2 out]
        "Ready?" <- FALSE ("Ready?")
      }
    }
    n538 = Unbundle By Name(w788) -> ("status"=w787:bool)
    n539 = Or(x=w787, y=w790) -> (x .or. y?=w789:bool)
  }
  n540 = local read "Sensitivity"() -> (w2:T4)
  n541 = case shown="\"-1V..1V\", Default" w2 {
    tunnel: [-1.0 ("maximum value") -1.25 ("maximum value") -2.0 ("maximum value") -2.5 ("maximum value") -4.0 ("maximum value") -5.0 ("maximum value") -10.0 ("maximum value")] -> _
    tunnel: [1.0 ("maximum value") 1.25 ("maximum value") 2.0 ("maximum value") 2.5 ("maximum value") 4.0 ("maximum value") 5.0 ("maximum value") 10.0 ("maximum value")] -> _
    frame "-1V..1V", Default {
    }
    frame "-1.25V..1.25V" {
    }
    frame "-2V..2V" {
    }
    frame "-2.5V..2.5V" {
    }
    frame "-4V..4V" {
    }
    frame "-5V..5V" {
    }
    frame "-10V..10V" {
    }
  }
  n542 = Merge Errors(w6, w5) -> (w4:errorcluster)
  n543 = Release Queue(queue=w7, error in (no error)=w4) -> ()  [unwired: 1 in, 3 out]
